vi "Fuel Injector Analysis Section.vi"(8 "error in (no error)":errorcluster, 11 "Node Ptr":T5 format="%.0x") -> (0 "error out":errorcluster)   [LabVIEW 2019, in "Fuel Injector Analysis Addon System Explorer.lvlib"]
uses:
  Fuel Injector Analysis Addon System Explorer.lvlib
  <vilib>/NI VeriStand/Custom Device API/Custom Device Item Ref.ctl
  Addon Shared/Types/Stage.PullIn.Types.ctl
  Addon Shared/Types/Stage.Transition.Types.ctl
  Types/Analysis.UI.Refs.ctl
  Addon Shared/Types/Analysis.Channels.Select.ctl
  <vilib>/NI VeriStand/Custom Device Tools/Custom Device Utility Library/Search Direction.ctl
  Addon Shared/SubVIs/Constants.vi
  <vilib>/NI VeriStand/Custom Device API/Set Item Property (U32).vi
  <vilib>/NI VeriStand/Custom Device API/Set Item Property (Variant).vi
  <vilib>/NI VeriStand/Custom Device API/Get Item Property (Variant).vi
  <vilib>/NI VeriStand/Custom Device API/Get Item Property (U32).vi
  <vilib>/NI VeriStand/Custom Device Tools/Custom Device Utility Library/NI VeriStand - Search for All Items by GUID.vi
  <vilib>/NI VeriStand/Custom Device Tools/Custom Device Utility Library/NI VeriStand - Search for Item by GUID.vi
  <vilib>/NI VeriStand/Custom Device API/Custom Device API.lvlib
  Addon Shared/Fuel Injector Analysis Addon Shared.lvlib
  <vilib>/NI VeriStand/Custom Device Tools/Custom Device Utility Library/Custom Device Utility Library.lvlib
panel:
  in  "Back":bool
  in  "Next":bool
  in  "Tab Control":T1(tab)
  in  "Path":path
  in  "Stages":string[](array[string])=["Boost", "Battery", "Off"]
  in  "Max Shots":T2(ring)=enum."1"
  out "Total Duration":dbl=1.0 caption="Total Event Duration" format="%#_p"
  in  "Pre-Trigger Samples":u8=1
  in  "Event Duration":dbl=1.0 format="%#_p"
  in  "Active Edge":bool=TRUE
  in  "Trigger Duration":dbl=1.0 caption="Trigger Duration (sec)" format="%#_p"
  in  "Initial Voltage Threshold":dbl=1.0 caption="Initial Voltage" format="%#_p"
  in  "Transitions":i32(listbox)
  in  "Pull In Type":T3
  in  "Stage Transition":T4
  in  "Level":dbl=1.0 format="%#_p"
  in  "Analysis":i32(listbox)=7
  in  "Stages List":i32(listbox)
  in  "Reset":bool
  in  "Apply":bool
  out "Injection":waveform(dbl)[](graph)
  out "Step":string
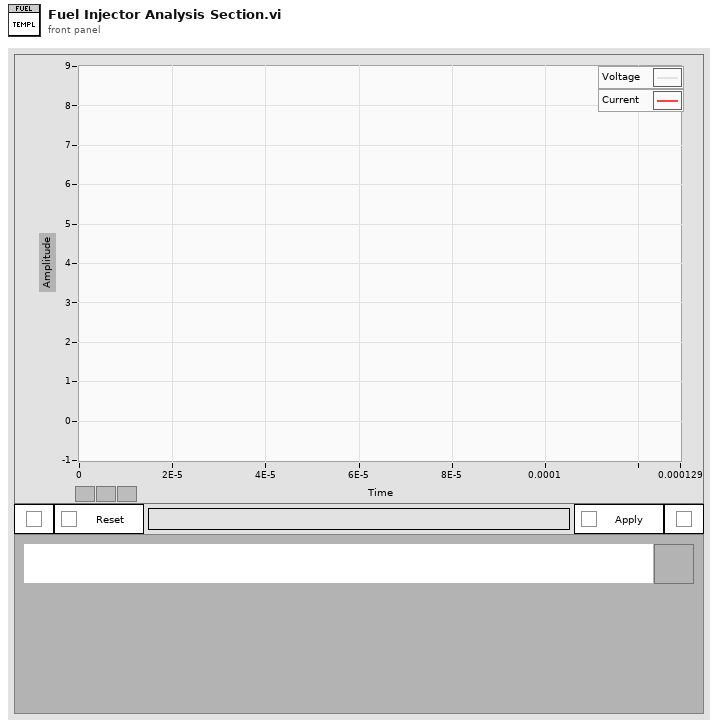
[diagram p1: front panel]
types:
  T1 = enum32{"Load Waveform", "Set Shots and Stages", "Set Event Duration", "Set Initial Voltage", "Set Stage Parsing Parameters", "Set Analysis Channels"}
  T2 = enum16{"0", "1", "2", "3", "4", "5", "6", "7", "8"}
  T3 = typedef "Fuel Injector Analysis Addon Shared.lvlib/Stage.PullIn.Types.ctl" = enum8{"Pull In Transition Pulses", "Pull In Transition Current Drop"}
  T4 = typedef "Fuel Injector Analysis Addon Shared.lvlib/Stage.Transition.Types.ctl" = enum8{"Stage Transition Inactive Time", "Stage Transition Voltage Increase", "Stage Transition Current Decrease", "Stage Transition Active Time"}
  T5 = typedef "Custom Device API.lvlib/Custom Device Item Ref.ctl" = u64
  T6 = typedef "Fuel Injector Analysis Addon System Explorer.lvlib/Analysis.UI.Refs.ctl" = cluster{"Path":refnum<vi>, "Pull In Transition":refnum<vi>, "Level":refnum<vi>, "Stage Transition":refnum<vi>, "Injection":refnum<vi>, "Tab":refnum<vi>, "Step":refnum<vi>, "Stages":refnum<vi>, "Transitions":refnum<vi>, "Initial Voltage":refnum<vi>, "Event Duration":refnum<vi>, "Max Shots":refnum<vi>, "Stages List":refnum<vi>, "Analysis":refnum<vi>, "Pre-Trigger Samples":refnum<vi>, "Trigger Duration":refnum<vi>, "dt":dbl, "Total Duration":refnum<vi>, "Next":refnum<vi>, "Back":refnum<vi>, "Active Edge":refnum<vi>}
  T7 = enum8{"Enabled", "Disabled", "Disabled and Grayed Out"}
  T8 = typedef "Fuel Injector Analysis Addon Shared.lvlib/Analysis.Channels.Select.ctl" = cluster{"Pull In Time":bool, "Pull In Max Current":bool, "Pull In Max Voltage":bool, "Pull In Min Voltage":bool, "Pull In Avg Voltage":bool, "Hold Time":bool, "Hold Max Current":bool, "Hold Min Current":bool, "Hold Avg Current":bool, "Hold Max Voltage":bool, "Hold Min Voltage":bool, "Hold Avg Max Voltage":bool, "Hold Avg Min Voltage":bool, "Off Time":bool, "Off Max Current":bool, "Off Min Current":bool, "Off Avg Current":bool, "Off Max Voltage":bool, "Off Min Voltage":bool, "Off Avg Voltage":bool, "Total Voltage Pulses":bool, "Total Stage Time":bool}
  T9 = typedef "Custom Device Utility Library.lvlib/Search Direction.ctl" = enum16{"Down", "Up"}
  T10 = typedef "Custom Device API.lvlib/Custom Device Commands.ctl" = enum16{"Default", "Item renamed", "Shutdown", "Dynamic button pressed"}
  T11 = typedef "LVPoint32TypeDef.ctl" = cluster{"Horizontal":i32, "Vertical":i32}
  T12 = typedef "LVCursorListTypeDef.ctl" = cluster{"Name":string, "Color":u32, "Style":u8, "Point Style":u8, "Name Visible":bool, "Allow Drag":bool, "Cursor Mode":u32, "Plot":i32, "Index":i32, "Position":cluster{"X":dbl, "Y":dbl}, "X Scale":u32, "Y Scale":u32, "Watch Plots":i32[], "Watch All Plots":bool, "Plot Area":i32, "Label Offset":cluster{"X":dbl, "Y":dbl}}[]
  T13 = cluster{"Name":string, "Color":u32, "Style":u8, "Point Style":u8, "Name Visible":bool, "Allow Drag":bool, "Cursor Mode":u32, "Plot":i32, "Index":i32, "Position":cluster{"X":dbl, "Y":dbl}, "X Scale":u32, "Y Scale":u32, "Watch Plots":i32[], "Watch All Plots":bool, "Plot Area":i32, "Label Offset":cluster{"X":dbl, "Y":dbl}}
  T14 = typedef "Custom Device API.lvlib/Custom Device Channel.ctl" = cluster{"Type":T15, "Units":string, "Default Value":dbl, "Faultable":bool, "Scalable":bool}
  T15 = typedef "Custom Device API.lvlib/Custom Device Channel Type.ctl" = enum16{"Input", "Output"}
  T16 = typedef "Custom Device API.lvlib/Custom Device Item Info.ctl" = cluster{"Name":string, "Is Channel":bool, "GUID":string, "Is Waveform":bool}
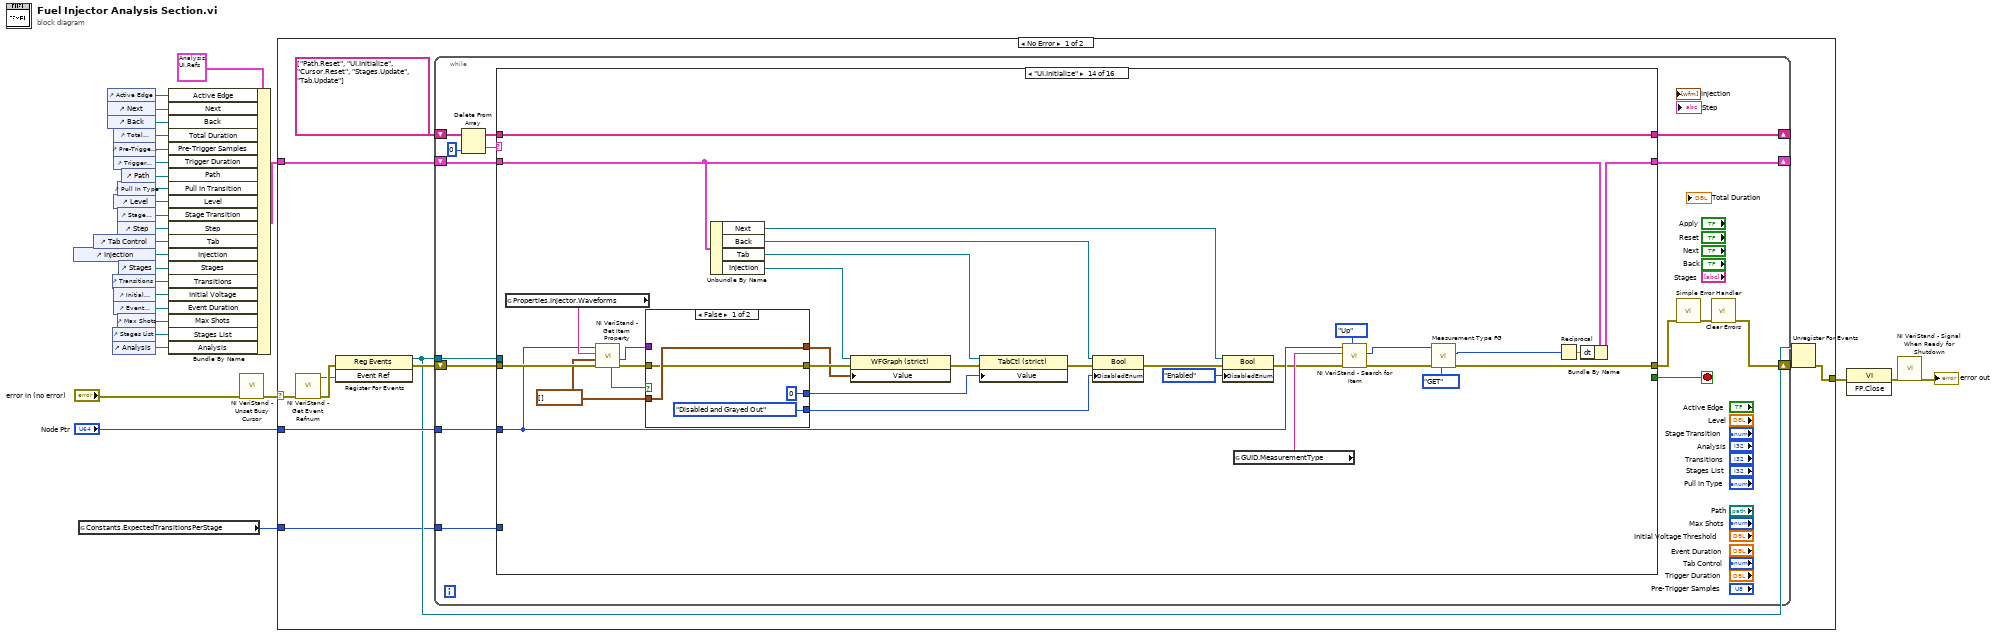
[diagram p0: block diagram]
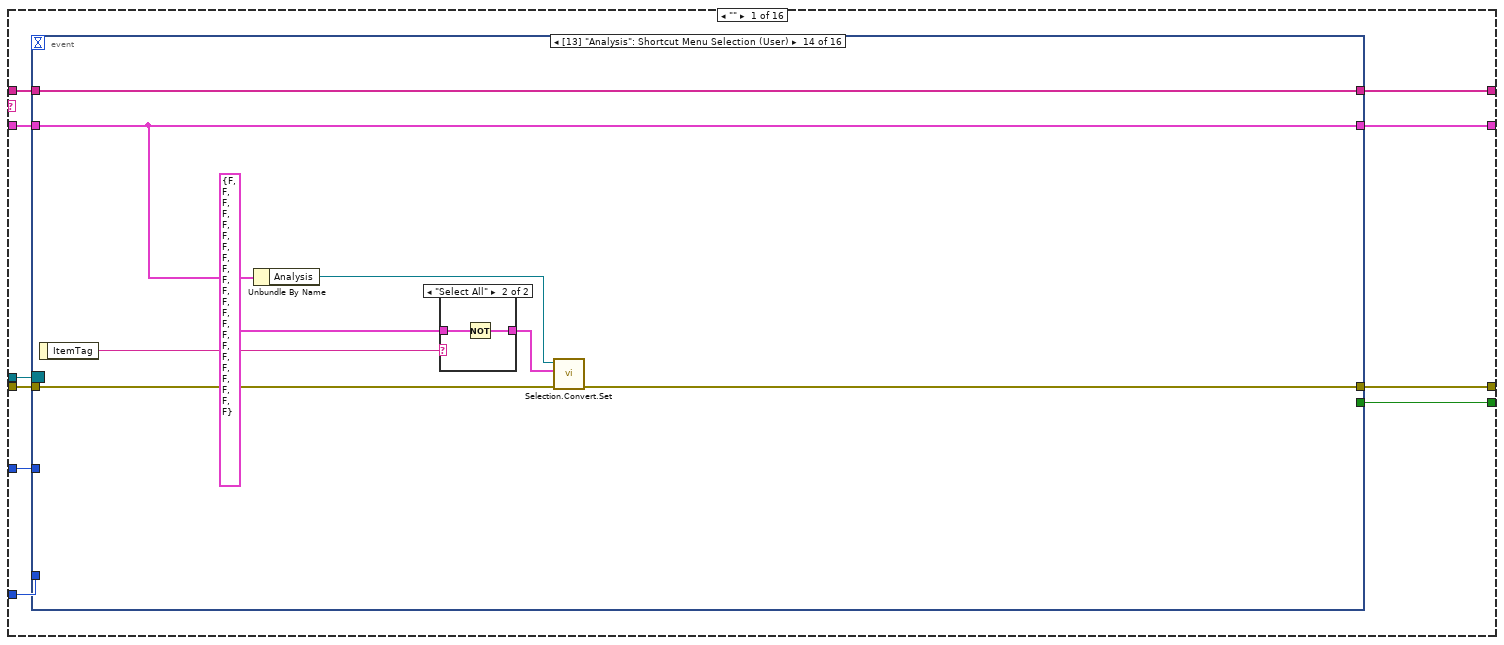
[diagram p2: hidden frame]
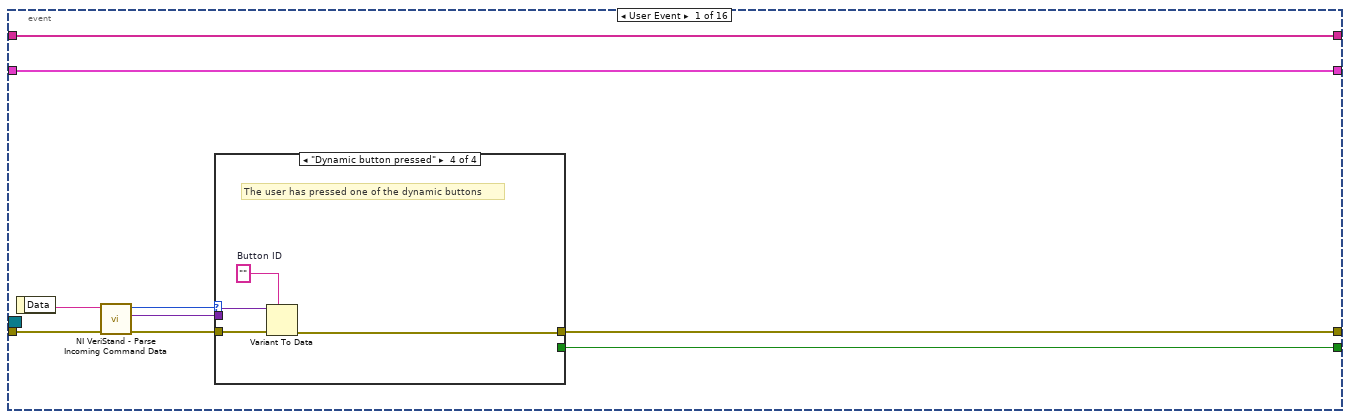
[diagram p3: hidden frame]
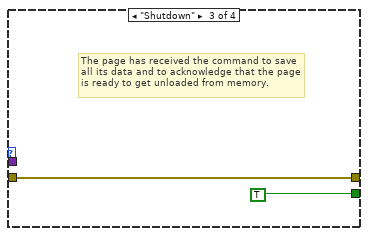
[diagram p6: hidden frame]
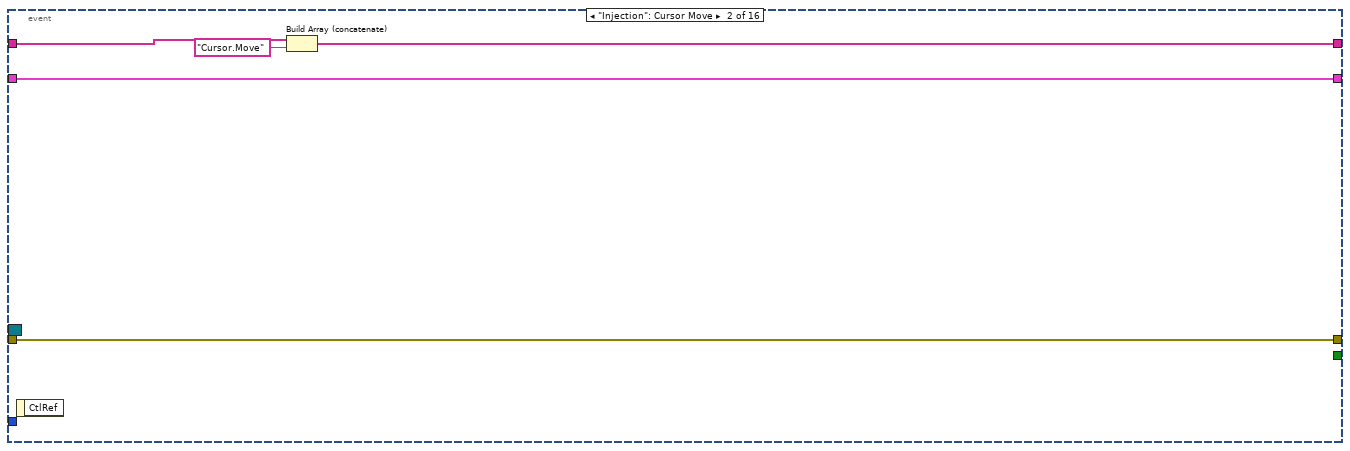
[diagram p7: hidden frame]
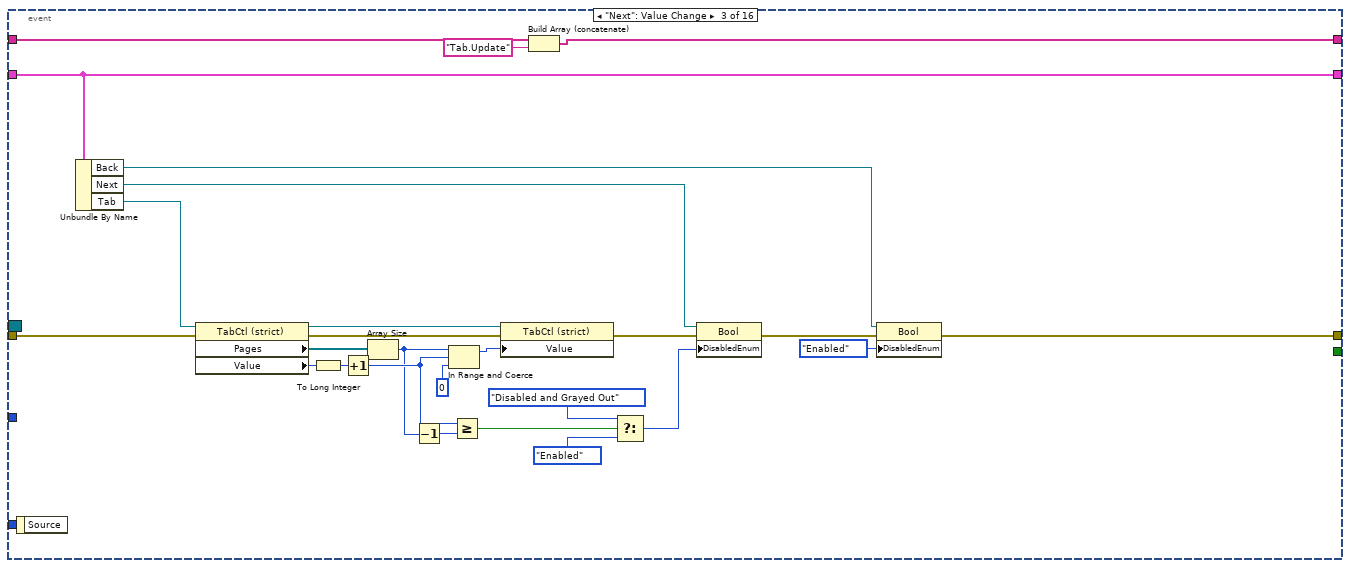
[diagram p8: hidden frame]
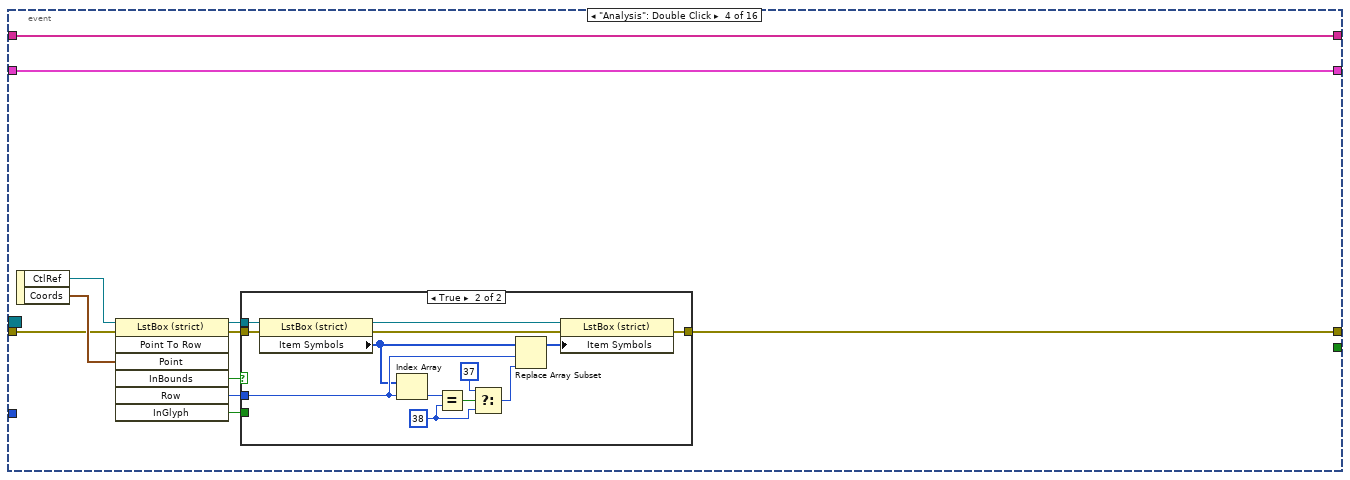
[diagram p9: hidden frame]
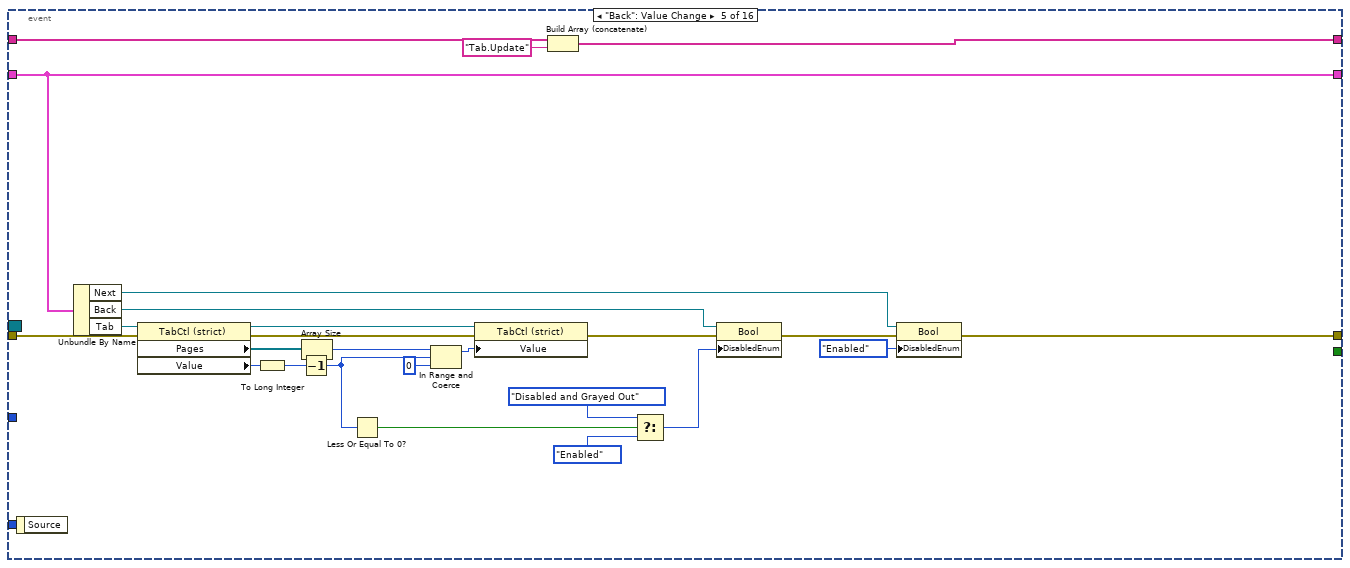
[diagram p11: hidden frame]
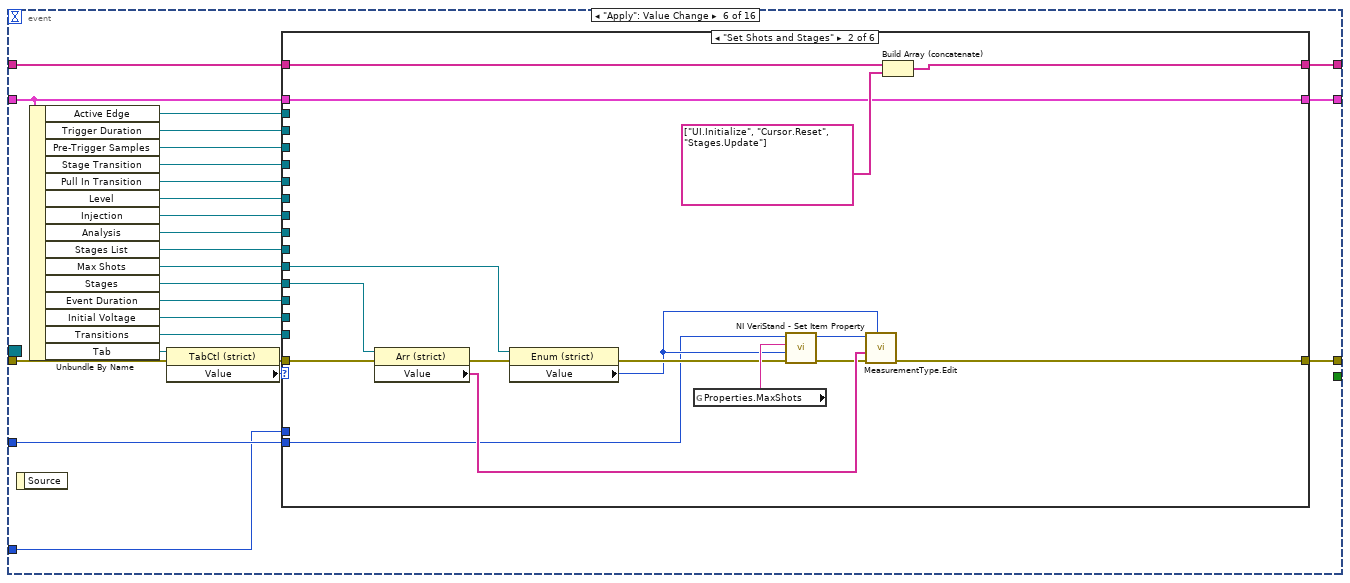
[diagram p12: hidden frame]
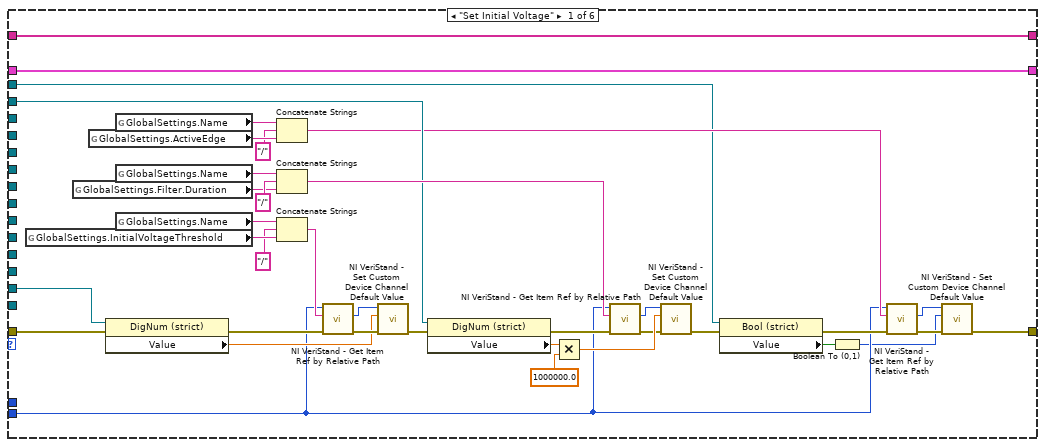
[diagram p13: hidden frame]
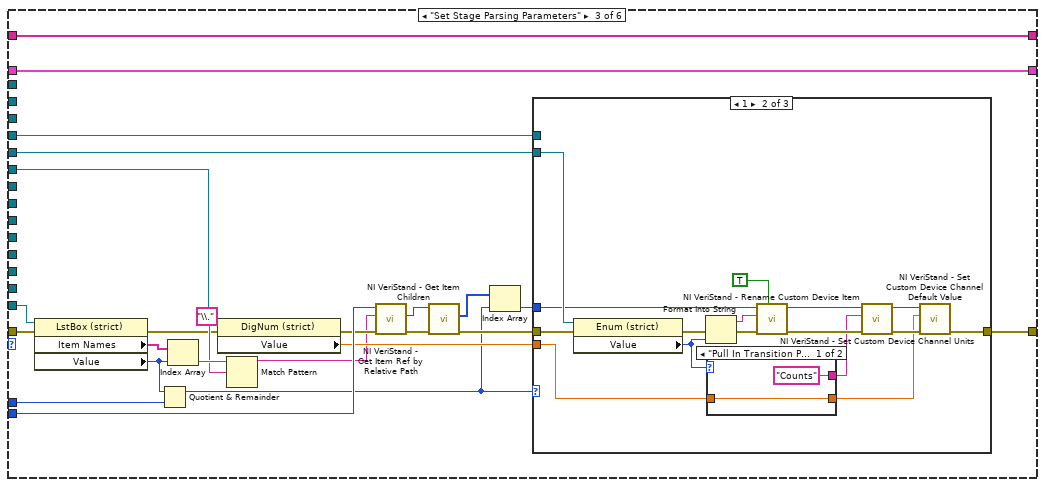
[diagram p14: hidden frame]
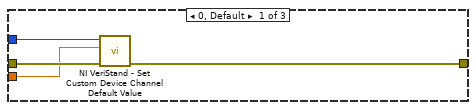
[diagram p15: hidden frame]
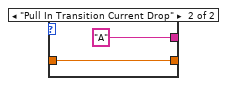
[diagram p16: hidden frame]
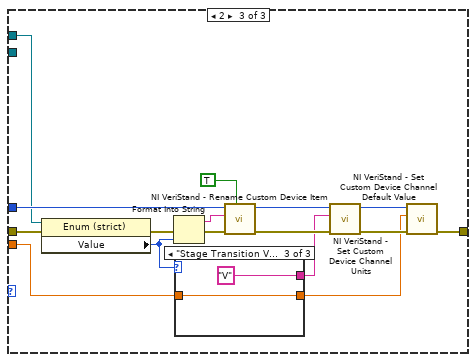
[diagram p17: hidden frame]
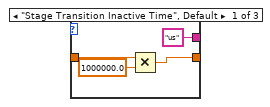
[diagram p18: hidden frame]
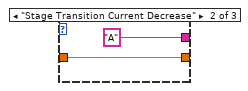
[diagram p19: hidden frame]
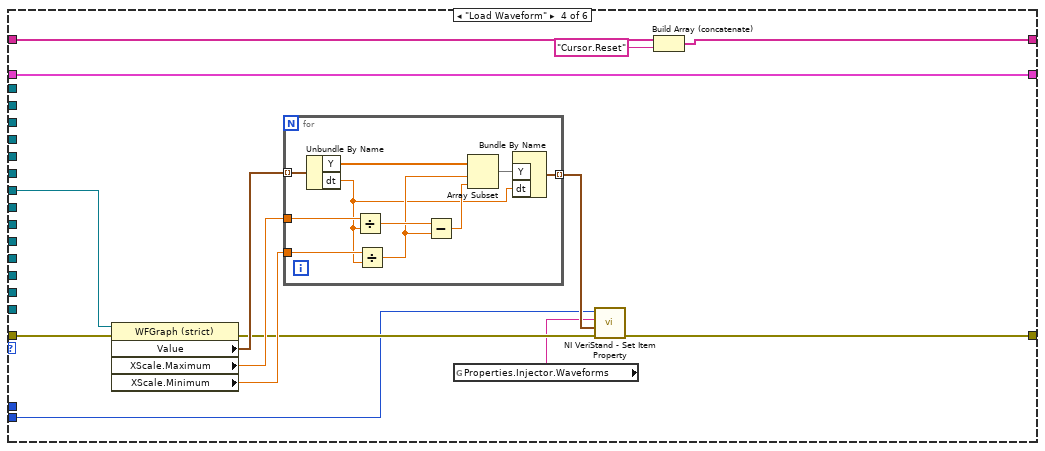
[diagram p20: hidden frame]
diagram:
  n1 = control-ref of="Injection"() -> (w21:refnum<vi>)
  n2 = global read "Constants.vi" "Constants.ExpectedTransitionsPerStage"() -> (w7:u32)
  n3 = control-ref of="Tab Control"() -> (w10:refnum<vi>)
  n4 = control-ref of="Active Edge"() -> (w1:refnum<vi>)
  n5 = control-ref of="Next"() -> (w3:refnum<vi>)
  n6 = control-ref of="Back"() -> (w2:refnum<vi>)
  n7 = control-ref of="Transitions"() -> (w16:refnum<vi>)
  n8 = control-ref of="Stages List"() -> (w12:refnum<vi>)
  n9 = control-ref of="Analysis"() -> (w11:refnum<vi>)
  n10 = control-ref of="Total Duration"() -> (w4:refnum<vi>)
  n11 = control-ref of="Pre-Trigger Samples"() -> (w5:refnum<vi>)
  n12 = control-ref of="Trigger Duration"() -> (w6:refnum<vi>)
  n13 = control-ref of="Level"() -> (w20:refnum<vi>)
  n14 = control-ref of="Initial Voltage Threshold"() -> (w15:refnum<vi>)
  n15 = control-ref of="Event Duration"() -> (w14:refnum<vi>)
  n16 = control-ref of="Pull In Type"() -> (w9:refnum<vi>)
  n17 = control-ref of="Stage Transition"() -> (w8:refnum<vi>)
  n18 = control-ref of="Step"() -> (w18:refnum<vi>)
  n19 = control-ref of="Max Shots"() -> (w13:refnum<vi>)
  n20 = control-ref of="Stages"() -> (w17:refnum<vi>)
  n21 = control-ref of="Path"() -> (w19:refnum<vi>)
  n22 = Bundle By Name(cluster=T6 {"Path"=refnum, "Pull In Transition"=refnum, "Level"=refnum, "Stage Transition"=refnum, "Injection"=refnum, "Tab"=refnum, "Step"=refnum, "Stages"=refnum, "Transitions"=refnum, "Initial Voltage"=refnum, "Event Duration"=refnum, "Max Shots"=refnum, "Stages List"=refnum, "Analysis"=refnum, "Pre-Trigger Samples"=refnum, "Trigger Duration"=refnum, "dt"=0.0, "Total Duration"=refnum, "Next"=refnum, "Back"=refnum, "Active Edge"=refnum}, "Active Edge"=w1, "Next"=w3, "Back"=w2, "Total Duration"=w4, "Pre-Trigger Samples"=w5, "Trigger Duration"=w6, "Path"=w19, "Pull In Transition"=w9, "Level"=w20, "Stage Transition"=w8, "Step"=w18, "Tab"=w10, "Injection"=w21, "Stages"=w17, "Transitions"=w16, "Initial Voltage"=w15, "Event Duration"=w14, "Max Shots"=w13, "Stages List"=w12, "Analysis"=w11) -> (w23:T6)
  n23 = call <vilib>:"NI VeriStand - Unset Busy Cursor.vi"("error in (no error)"="error in (no error)") -> ("error out"=w25:errorcluster)  [unwired: 10 out]
  n24 = case shown="No Error" w25 {
    selector: w25 -> [w34 w1059]
    tunnel: [w38 w1057] -> w29
    tunnel: "Node Ptr" -> [w35 _]
    tunnel: w23 -> [w33 _]
    tunnel: w7 -> [w30 _]
    frame No Error {
      n25 = call <vilib>:"NI VeriStand - Get Event Refnum.vi"("error in (no error)"=w34) -> ("error out"=w40:errorcluster, "Event Ref"=w37:refnum<user-event>)  [unwired: 9 out]
      n26 = register-events(error in=w40, w37) -> (reference out=w31:refnum<event-registration>, error out=w36:errorcluster)  [unwired: 1 in]
      n27 = while {
        tunnel: w35 -> [w53]
        shift-right: [w50] -> w39
        shift-left: w36 -> [w55]
        shift-right: [w43] -> _
        shift-left: string[] ["Path.Reset", "UI.Initialize", "Cursor.Reset", "Stages.Update", "Tab.Update"] -> [w48]
        tunnel: w31 -> [w44]
        tunnel: w30 -> [w42]
        shift-right: [w41] -> _
        shift-left: w33 -> [w49]
        stop <- w54 stop-if-true
        n28 = Delete From Array(array=w48, index=0) -> (deleted portion=w46:string, array with subset deleted=w45:string[])  [unwired: 1 in]
        n29 = case shown="\"UI.Initialize\"" w46 {
          tunnel: w55 -> [w65 w470 w505 w632 w645 w659 w676 w716 w760 w776 w811 w855 w878 w1029 w1050 w1056]
          tunnel: w44 -> [w64 _ _ _ _ _ _ _ _ _ _ _ _ _ _ _]
          tunnel: [w63 _ _ _ _ _ _ _ _ _ _ _ _ _ _ _] -> w54
          tunnel: w53 -> [w62 w469 w498 _ _ _ w677 w693 w744 w774 _ _ w877 w1022 _ _]
          tunnel: [w61 w471 w503 w633 w644 w658 w673 w696 w734 w770 w819 w854 w876 w1018 w1050 w1053] -> w52
          tunnel: w49 -> [w60 w472 w504 w640 w647 w661 w684 w715 w759 w791 w805 w866 w868 w1015 w1048 w1054]
          tunnel: w45 -> [w59 w481 w495 w634 w653 w667 w672 w707 w767 w787 w817 w867 w874 w1027 w1049 w1055]
          tunnel: [w58 w481 w494 w634 w653 w667 w672 w706 w754 w787 w818 w867 w873 w1027 w1049 w1055] -> w43
          tunnel: w42 -> [w57 _ w497 _ _ _ _ _ _ _ _ _ w871 _ _ _]
          tunnel: [w56 w472 w504 w640 w647 w661 w684 w715 w759 w791 w806 w866 w869 w1014 w1048 w1054] -> w41
          frame "" {
            n30 = event shown="[13] \"Analysis\": Shortcut Menu Selection (User)" {
              selector: w64 -> [_ _ _ _ _ _ _ _ _ _ _ _ _ _ _ _]
              dyn-events: _ -> [_ _ _ _ _ _ _ _ _ _ _ _ _ _ _ _]
              timeout: _ -> [_ _ _ _ _ _ _ _ _ _ _ _ _ _ _ _]
              tunnel: w65 -> [w74 w84 w113 w116 w163 w188 w380 w387 w390 w395 w404 w417 w440 w453 w460 w465]
              tunnel: [w70 _ _ _ _ _ _ _ _ _ _ _ _ _ _ _] -> w63
              tunnel: [w69 w84 w98 w115 w145 w182 w380 w387 w390 w395 w402 w413 w439 w450 w460 w465] -> w61
              tunnel: w62 -> [_ _ _ _ _ w183 _ _ _ _ _ _ _ _ _ _]
              tunnel: w60 -> [w66 w83 w108 w114 w158 w165 w379 w384 w389 w394 w405 w418 w431 w452 w461 w466]
              tunnel: w59 -> [w67 w87 w105 w124 w156 w177 w383 w388 w393 w398 w400 w415 w435 w454 w462 w467]
              tunnel: [w67 w86 w104 w124 w155 w176 w382 w386 w392 w397 w399 w414 w434 w454 w459 w464] -> w58
              tunnel: w57 -> [_ _ _ _ _ w169 _ _ _ _ _ _ _ _ _ _]
              tunnel: [w66 w83 w108 w114 w158 w166 w379 w384 w389 w394 w405 w418 w431 w452 w461 w466] -> w56
              event User Event {
                n31 = event-data() -> ("Data"=w73:string)  [unwired: 1 out]
                n32 = call <vilib>:"NI VeriStand - Parse Incoming Command Data.vi"("error in (no error)"=w74, "Incoming data"=w73) -> ("error out"=w72:errorcluster, "Outgoing data"=w68:variant, "Action"=w71:T10)  [unwired: 7 out]
                n33 = case shown="\"Dynamic button pressed\"" w71 {
                  tunnel: w72 -> [w75 w76 w77 w82]
                  tunnel: [_ _ TRUE _] -> w70
                  tunnel: [w75 w76 w77 w79] -> w69
                  tunnel: w68 -> [_ _ _ w81]
                  frame "Default", Default {
                  }
                  frame "Item renamed" {
                  }
                  frame "Shutdown" {
                    # "The page has received the command to save all its data and to acknowledge that the page is ready to get unloaded from memory."
                  }
                  frame "Dynamic button pressed" {
                    w80 = ""  # Button ID
                    # "The user has pressed one of the dynamic buttons"
                    n34 = Variant To Data(error in=w82, type=w80, Variant=w81) -> (error out=w79:errorcluster)  [unwired: 1 out]
                  }
                }
              }
              event "Injection": Cursor Move {
                n35 = event-data() -> ()  [unwired: 2 out]
                n36 = Build Array (concatenate)(w87, "Cursor.Move") -> (w86:string[])
              }
              event "Next": Value Change {
                n37 = event-data() -> ()  [unwired: 2 out]
                n38 = Unbundle By Name(w108) -> ("Back"=w96:refnum<vi>, "Next"=w97:refnum<vi>, "Tab"=w107:refnum<vi>)
                n39 = property class="TabCtl (strict)"(reference=w107, error in=w113) -> (reference out=w110:refnum<vi>, error out=w103:errorcluster, "Pages"=w112:refnum<vi>[], "Value"=w111:T1)
                n40 = To Long Integer(number=w111) -> (32bit integer=w102:i32)
                n41 = Increment(x=w102) -> (x+1=w90:i32)
                n42 = Array Size(array=w112) -> (size(s)=w89:i32)
                n43 = Decrement(x=w89) -> (x-1=w88:i32)
                n44 = In Range and Coerce(upper limit=w89, x=w90, lower limit=0) -> (coerced(x)=w109:i32)  [unwired: 1 out]
                n45 = Greater Or Equal?(x=w90, y=w88) -> (x >= y?=w94:bool)
                n46 = property class="TabCtl (strict)"(reference=w110, error in=w103, "Value"=w109) -> (error out=w99:errorcluster)  [unwired: 1 out]
                n47 = Build Array (concatenate)(w105, "Tab.Update") -> (w104:string[])
                n48 = Select(t=T7."Disabled and Grayed Out" ("Disabled"), s=w94, f=T7."Enabled" ("Disabled")) -> (s? t:f=w91:T7)
                n49 = property class="Bool"(reference=w97, error in=w99, "DisabledEnum"=w91) -> (error out=w100:errorcluster)  [unwired: 1 out]
                n50 = property class="Bool"(reference=w96, error in=w100, "DisabledEnum"=T7."Enabled" ("Disabled")) -> (error out=w98:errorcluster)  [unwired: 1 out]
              }
              event "Analysis": Double Click {
                n51 = event-data() -> ("CtlRef"=w118:refnum<vi>, "Coords"=w117:T11)  [unwired: 1 out]
                n52 = invoke class="LstBox (strict)" method="Point To Row"(reference=w118, error in=w116, "Point"=w117) -> (reference out=w122:refnum<vi>, error out=w121:errorcluster, "InBounds"=w119:bool, "Row"=w120:i32, "InGlyph"=w123:bool)  [unwired: 4 in, 2 out]
                n53 = case shown="True" w119 {
                  tunnel: w123 -> [_ _]
                  tunnel: w122 -> [_ w138]
                  tunnel: w121 -> [w125 w137]
                  tunnel: w120 -> [_ w136]
                  tunnel: [w125 w126] -> w115
                  frame False {
                  }
                  frame True {
                    w133 = 38
                    n54 = property class="LstBox (strict)"(reference=w138, error in=w137) -> (reference out=w129:refnum<vi>, error out=w128:errorcluster, "Item Symbols"=w131:i32[])
                    n55 = Index Array(array=w131, index=w136) -> (element=w135:i32)
                    n56 = Equal?(x=w135, y=w133) -> (x = y?=w134:bool)
                    n57 = Select(t=37, s=w134, f=w133) -> (s? t:f=w130:i32)
                    n58 = Replace Array Subset(array=w131, new element=w130, index=w136) -> (w127:i32[])
                    n59 = property class="LstBox (strict)"(reference=w129, error in=w128, "Item Symbols"=w127) -> (error out=w126:errorcluster)  [unwired: 1 out]
                  }
                }
              }
              event "Back": Value Change {
                n60 = event-data() -> ()  [unwired: 2 out]
                n61 = Unbundle By Name(w158) -> ("Next"=w143:refnum<vi>, "Back"=w144:refnum<vi>, "Tab"=w157:refnum<vi>)
                n62 = property class="TabCtl (strict)"(reference=w157, error in=w163) -> (reference out=w160:refnum<vi>, error out=w153:errorcluster, "Pages"=w162:refnum<vi>[], "Value"=w161:T1)
                n63 = To Long Integer(number=w161) -> (32bit integer=w152:i32)
                n64 = Decrement(x=w152) -> (x-1=w140:i32)
                n65 = Array Size(array=w162) -> (size(s)=w141:i32)
                n66 = Less Or Equal To 0?(x=w140) -> (x <= 0?=w139:bool)
                n67 = In Range and Coerce(upper limit=w141, x=w140, lower limit=0) -> (coerced(x)=w159:i32)  [unwired: 1 out]
                n68 = property class="TabCtl (strict)"(reference=w160, error in=w153, "Value"=w159) -> (error out=w146:errorcluster)  [unwired: 1 out]
                n69 = Build Array (concatenate)(w156, "Tab.Update") -> (w155:string[])
                n70 = Select(t=T7."Disabled and Grayed Out" ("Disabled"), s=w139, f=T7."Enabled" ("Disabled")) -> (s? t:f=w147:T7)
                n71 = property class="Bool"(reference=w144, error in=w146, "DisabledEnum"=w147) -> (error out=w151:errorcluster)  [unwired: 1 out]
                n72 = property class="Bool"(reference=w143, error in=w151, "DisabledEnum"=T7."Enabled" ("Disabled")) -> (error out=w145:errorcluster)  [unwired: 1 out]
              }
              event "Apply": Value Change {
                n73 = event-data() -> ()  [unwired: 2 out]
                n74 = Unbundle By Name(w165) -> ("Active Edge"=w164:refnum<vi>, "Trigger Duration"=w167:refnum<vi>, "Pre-Trigger Samples"=w168:refnum<vi>, "Stage Transition"=w172:refnum<vi>, "Pull In Transition"=w173:refnum<vi>, "Level"=w174:refnum<vi>, "Injection"=w175:refnum<vi>, "Analysis"=w178:refnum<vi>, "Stages List"=w179:refnum<vi>, "Max Shots"=w180:refnum<vi>, "Stages"=w181:refnum<vi>, "Event Duration"=w184:refnum<vi>, "Initial Voltage"=w185:refnum<vi>, "Transitions"=w170:refnum<vi>, "Tab"=w187:refnum<vi>)
                n75 = property class="TabCtl (strict)"(reference=w187, error in=w188) -> (error out=w186:errorcluster, "Value"=w171:T1)  [unwired: 1 out]
                n76 = case shown="\"Set Shots and Stages\"" w171 {
                  tunnel: w186 -> [w222 w241 w264 w327 w352 w354]
                  tunnel: w185 -> [w221 _ _ _ _ _]
                  tunnel: [w193 w231 w256 w320 w341 w355] -> w182
                  tunnel: w184 -> [_ _ _ _ _ w375]
                  tunnel: w183 -> [w191 w230 w260 w318 w348 w360]
                  tunnel: w181 -> [_ w238 _ _ _ _]
                  tunnel: w180 -> [_ w237 _ _ _ _]
                  tunnel: w179 -> [_ _ _ _ w351 _]
                  tunnel: w178 -> [_ _ _ _ w343 _]
                  tunnel: w177 -> [w215 w236 w265 w326 w340 w369]
                  tunnel: [w215 w235 w265 w316 w340 w369] -> w176
                  tunnel: w175 -> [_ _ _ w325 _ _]
                  tunnel: w174 -> [_ _ w253 _ _ _]
                  tunnel: w173 -> [_ _ w251 _ _ _]
                  tunnel: w172 -> [_ _ w250 _ _ _]
                  tunnel: w170 -> [_ _ w244 _ _ _]
                  tunnel: w169 -> [_ _ w243 _ _ _]
                  tunnel: w168 -> [_ _ _ _ _ w358]
                  tunnel: w167 -> [w207 _ _ _ _ _]
                  tunnel: [w203 w228 w242 w314 w338 w356] -> w166
                  tunnel: w165 -> [w203 w228 w242 w314 w338 w356]
                  tunnel: w164 -> [w190 _ _ _ _ _]
                  frame "Set Initial Voltage" {
                    n77 = global read "Constants.vi" "GlobalSettings.InitialVoltageThreshold"() -> (w224:string)
                    n78 = global read "Constants.vi" "GlobalSettings.Filter.Duration"() -> (w210:string)
                    n79 = global read "Constants.vi" "GlobalSettings.ActiveEdge"() -> (w201:string)
                    n80 = property class="DigNum (strict)"(reference=w221, error in=w222) -> (error out=w218:errorcluster, "Value"=w217:dbl)  [unwired: 1 out]
                    n81 = global read "Constants.vi" "GlobalSettings.Name"() -> (w202:string)
                    n82 = global read "Constants.vi" "GlobalSettings.Name"() -> (w209:string)
                    n83 = global read "Constants.vi" "GlobalSettings.Name"() -> (w225:string)
                    n84 = Concatenate Strings(w202, "/" ("string"), w201) -> (w192:string)
                    n85 = Concatenate Strings(w209, "/" ("string"), w210) -> (w214:string)
                    n86 = Concatenate Strings(w225, "/" ("string"), w224) -> (w216:string)
                    n87 = call <vilib>:"NI VeriStand - Get Item Ref by Relative Path.vi"("error in"=w218, "Relative Item Path"=w216, "Section Ref in"=w191) -> ("error out"=w220:errorcluster, "Item Ref"=w219:T5)  [unwired: 5 in, 2 out]
                    n88 = call <vilib>:"NI VeriStand - Set Custom Device Channel Default Value.vi"("error in (no error)"=w220, "Default Value"=w217, "Channel Ref in"=w219) -> ("error out"=w208:errorcluster)  [unwired: 7 in, 1 out]
                    n89 = property class="DigNum (strict)"(reference=w207, error in=w208) -> (error out=w213:errorcluster, "Value"=w205:dbl)  [unwired: 1 out]
                    n90 = Multiply(x=w205, y=1000000.0) -> (x*y=w204:dbl)
                    n91 = call <vilib>:"NI VeriStand - Get Item Ref by Relative Path.vi"("error in"=w213, "Relative Item Path"=w214, "Section Ref in"=w191) -> ("error out"=w196:errorcluster, "Item Ref"=w212:T5)  [unwired: 5 in, 2 out]
                    n92 = call <vilib>:"NI VeriStand - Set Custom Device Channel Default Value.vi"("error in (no error)"=w196, "Default Value"=w204, "Channel Ref in"=w212) -> ("error out"=w195:errorcluster)  [unwired: 7 in, 1 out]
                    n93 = property class="Bool (strict)"(reference=w190, error in=w195) -> (error out=w194:errorcluster, "Value"=w199:bool)  [unwired: 1 out]
                    n94 = Boolean To (0,1)(Boolean=w199) -> (0, 1=w189:i16)
                    n95 = call <vilib>:"NI VeriStand - Get Item Ref by Relative Path.vi"("error in"=w194, "Relative Item Path"=w192, "Section Ref in"=w191) -> ("error out"=w197:errorcluster, "Item Ref"=w198:T5)  [unwired: 5 in, 2 out]
                    n96 = call <vilib>:"NI VeriStand - Set Custom Device Channel Default Value.vi"("error in (no error)"=w197, "Default Value"=w189, "Channel Ref in"=w198) -> ("error out"=w193:errorcluster)  [unwired: 7 in, 1 out]
                  }
                  frame "Set Shots and Stages" {
                    n97 = property class="Arr (strict)"(reference=w238, error in=w241) -> (error out=w240:errorcluster, "Value"=w239:string[])  [unwired: 1 out]
                    n98 = property class="Enum (strict)"(reference=w237, error in=w240) -> (error out=w233:errorcluster, "Value"=w232:T2)  [unwired: 1 out]
                    n99 = global read "Constants.vi" "Properties.MaxShots"() -> (w234:string)
                    n100 = call-poly <vilib>:"NI VeriStand - Set Item Property.vi"("error in (no error)"=w233, "Value"=w232, "Property Name"=w234, "Item Ref in"=w230) -> ("error out"=w227:errorcluster, "Item Ref out"=w226:T5)  [unwired: 5 in, 1 out]
                    n101 = call "MeasurementType.Edit.vi"("Max Shots"=w232, "error in (no error)"=w227, "Stages"=w239, "Item Ref in"=w226) -> ("error out"=w231:errorcluster)  [unwired: 7 in]
                    n102 = Build Array (concatenate)(w236, string[] ["UI.Initialize", "Cursor.Reset", "Stages.Update"]) -> (w235:string[])
                  }
                  frame "Set Stage Parsing Parameters" {
                    n103 = property class="LstBox (strict)"(reference=w244, error in=w264) -> (error out=w255:errorcluster, "Item Names"=w263:string[], "Value"=w252:i32)  [unwired: 1 out]
                    n104 = Quotient & Remainder(x=w252, y=w243) -> (x-y*floor(x/y)=w246:u32)  [unwired: 1 out]
                    n105 = Index Array(array=w263, index=w252) -> (element=w262:string)
                    n106 = property class="DigNum (strict)"(reference=w253, error in=w255) -> (error out=w254:errorcluster, "Value"=w247:dbl)  [unwired: 1 out]
                    n107 = Match Pattern(string=w262, regular expression="\\.") -> (before substring=w245:string)  [unwired: 1 in, 3 out]
                    n108 = call <vilib>:"NI VeriStand - Get Item Ref by Relative Path.vi"("error in"=w254, "Relative Item Path"=w245, "Section Ref in"=w260) -> ("error out"=w259:errorcluster, "Item Ref"=w258:T5)  [unwired: 5 in, 2 out]
                    n109 = call <vilib>:"NI VeriStand - Get Item Children.vi"("error in (no error)"=w259, "Item Ref in"=w258) -> ("error out"=w249:errorcluster, "Child Refs"=w257:T5[])  [unwired: 6 in, 2 out]
                    n110 = Index Array(array=w257, index=w246) -> (element=w248:T5)
                    n111 = case shown="1" w246 {
                      tunnel: w249 -> [w269 w278 w305]
                      tunnel: [w267 w276 w294] -> w256
                      tunnel: w248 -> [w268 w271 w301]
                      tunnel: w251 -> [_ w285 _]
                      tunnel: w250 -> [_ _ w296]
                      tunnel: w247 -> [w266 w273 w291]
                      frame 0, Default {
                        n112 = call <vilib>:"NI VeriStand - Set Custom Device Channel Default Value.vi"("error in (no error)"=w269, "Default Value"=w266, "Channel Ref in"=w268) -> ("error out"=w267:errorcluster)  [unwired: 7 in, 1 out]
                      }
                      frame 1 {
                        n113 = property class="Enum (strict)"(reference=w285, error in=w278) -> (error out=w284:errorcluster, "Value"=w280:T3)  [unwired: 1 out]
                        n114 = Format Into String(error in=w284, w280) -> (resulting string=w270:string, error out=w283:errorcluster)  [unwired: 2 in]
                        n115 = case shown="\"Pull In Transition Pulses\", Default" w280 {
                          tunnel: ["Counts" "A"] -> w279
                          tunnel: [w286 w288] -> w274
                          tunnel: w273 -> [w286 w288]
                          frame "Pull In Transition Pulses", Default {
                          }
                          frame "Pull In Transition Current Drop" {
                          }
                        }
                        n116 = call <vilib>:"NI VeriStand - Rename Custom Device Item.vi"("Force Rename (F)"=TRUE, "error in (no error)"=w283, "New Name"=w270, "Item Ref in"=w271) -> ("error out"=w282:errorcluster, "Item Ref out"=w281:T5)  [unwired: 5 in, 1 out]
                        n117 = call <vilib>:"NI VeriStand - Set Custom Device Channel Units.vi"("error in (no error)"=w282, "Units"=w279, "Channel Ref in"=w281) -> ("error out"=w277:errorcluster, "Channel Ref out"=w275:T5)  [unwired: 7 in]
                        n118 = call <vilib>:"NI VeriStand - Set Custom Device Channel Default Value.vi"("error in (no error)"=w277, "Default Value"=w274, "Channel Ref in"=w275) -> ("error out"=w276:errorcluster)  [unwired: 7 in, 1 out]
                      }
                      frame 2 {
                        n119 = property class="Enum (strict)"(reference=w296, error in=w305) -> (error out=w304:errorcluster, "Value"=w298:T4)  [unwired: 1 out]
                        n120 = Format Into String(error in=w304, w298) -> (resulting string=w303:string, error out=w302:errorcluster)  [unwired: 2 in]
                        n121 = case shown="\"Stage Transition Voltage Increase\"" w298 {
                          tunnel: ["us" "A" "V"] -> w297
                          tunnel: [w307 w310 w312] -> w292
                          tunnel: w291 -> [w308 w310 w312]
                          frame "Stage Transition Inactive Time", Default {
                            n122 = Multiply(x=w308, y=1000000.0) -> (x*y=w307:dbl)
                          }
                          frame "Stage Transition Current Decrease" {
                          }
                          frame "Stage Transition Voltage Increase" {
                          }
                        }
                        n123 = call <vilib>:"NI VeriStand - Rename Custom Device Item.vi"("Force Rename (F)"=TRUE, "error in (no error)"=w302, "New Name"=w303, "Item Ref in"=w301) -> ("error out"=w300:errorcluster, "Item Ref out"=w299:T5)  [unwired: 5 in, 1 out]
                        n124 = call <vilib>:"NI VeriStand - Set Custom Device Channel Units.vi"("error in (no error)"=w300, "Units"=w297, "Channel Ref in"=w299) -> ("error out"=w295:errorcluster, "Channel Ref out"=w293:T5)  [unwired: 7 in]
                        n125 = call <vilib>:"NI VeriStand - Set Custom Device Channel Default Value.vi"("error in (no error)"=w295, "Default Value"=w292, "Channel Ref in"=w293) -> ("error out"=w294:errorcluster)  [unwired: 7 in, 1 out]
                      }
                    }
                  }
                  frame "Load Waveform" {
                    n126 = property class="WFGraph (strict)"(reference=w325, error in=w327) -> (error out=w321:errorcluster, "Value"=w324:waveform(dbl)[], "XScale.Maximum"=w323:dbl, "XScale.Minimum"=w322:dbl)  [unwired: 1 out]
                    n127 = for {
                      tunnel: w324 -> [w337] mode=indexing
                      tunnel: w323 -> [w336]
                      tunnel: w322 -> [w335]
                      tunnel: [w328] -> w319 mode=indexing
                      n128 = Unbundle By Name(w337) -> ("Y"=w333:dbl[], "dt"=w329:dbl)
                      n129 = Divide(x=w336, y=w329) -> (x/y=w334:dbl)
                      n130 = Divide(x=w335, y=w329) -> (x/y=w332:dbl)
                      n131 = Subtract(x=w334, y=w332) -> (x-y=w331:dbl)
                      n132 = Array Subset(array=w333, index=w332, length=w331) -> (w330:dbl[])
                      n133 = Bundle By Name("Y"=w330, "dt"=w329) -> (w328:waveform(dbl))  [unwired: 1 in]
                    }
                    n134 = global read "Constants.vi" "Properties.Injector.Waveforms"() -> (w317:string)
                    n135 = call-poly <vilib>:"NI VeriStand - Set Item Property.vi"("error in (no error)"=w321, "Value"=w319, "Property Name"=w317, "Item Ref in"=w318) -> ("error out"=w320:errorcluster)  [unwired: 5 in, 2 out]
                    n136 = Build Array (concatenate)(w326, "Cursor.Reset") -> (w316:string[])
                  }
                  frame "Set Analysis Channels" {
                    n137 = property class="LstBox (strict)"(reference=w351, error in=w352) -> (error out=w345:errorcluster, "Item Names"=w350:string[], "Value"=w349:i32)  [unwired: 1 out]
                    n138 = call "Selection.Convert.Get.vi"("error in (no error)"=w345, "ListBox in"=w343) -> ("error out"=w344:errorcluster, "Analysis Options"=w342:T8)  [unwired: 8 in]
                    n139 = Index Array(array=w350, index=w349) -> (element=w339:string)
                    n140 = call <vilib>:"NI VeriStand - Get Item Ref by Relative Path.vi"("error in"=w344, "Relative Item Path"=w339, "Section Ref in"=w348) -> ("error out"=w347:errorcluster, "Item Ref"=w346:T5)  [unwired: 5 in, 2 out]
                    n141 = call "Analysis.Selection.Create.vi"("error in (no error)"=w347, "Name"=w339, "Analysis Options"=w342, "Item Ref in"=w346) -> ("error out"=w341:errorcluster)  [unwired: 7 in]
                  }
                  frame "Set Event Duration" {
                    n142 = global read "Constants.vi" "GlobalSettings.PreTrigger.Samples"() -> (w362:string)
                    n143 = property class="DigNum (strict)"(reference=w358, error in=w354) -> (error out=w359:errorcluster, "Value"=w357:u8)  [unwired: 1 out]
                    n144 = global read "Constants.vi" "GlobalSettings.InjectionDuration"() -> (w377:string)
                    n145 = global read "Constants.vi" "GlobalSettings.Name"() -> (w378:string)
                    n146 = global read "Constants.vi" "GlobalSettings.Name"() -> (w361:string)
                    n147 = Concatenate Strings(w378, "/" ("string"), w377) -> (w370:string)
                    n148 = Concatenate Strings(w361, "/" ("string"), w362) -> (w366:string)
                    n149 = call <vilib>:"NI VeriStand - Get Item Ref by Relative Path.vi"("error in"=w359, "Relative Item Path"=w366, "Section Ref in"=w360) -> ("error out"=w364:errorcluster, "Item Ref"=w365:T5)  [unwired: 5 in, 2 out]
                    n150 = call <vilib>:"NI VeriStand - Set Custom Device Channel Default Value.vi"("error in (no error)"=w364, "Default Value"=w357, "Channel Ref in"=w365) -> ("error out"=w353:errorcluster)  [unwired: 7 in, 1 out]
                    n151 = property class="DigNum (strict)"(reference=w375, error in=w353) -> (error out=w372:errorcluster, "Value"=w371:dbl)  [unwired: 1 out]
                    n152 = call <vilib>:"NI VeriStand - Get Item Ref by Relative Path.vi"("error in"=w372, "Relative Item Path"=w370, "Section Ref in"=w360) -> ("error out"=w374:errorcluster, "Item Ref"=w373:T5)  [unwired: 5 in, 2 out]
                    n153 = Multiply(x=w371, y=1000000.0) -> (x*y=w368:dbl)
                    n154 = call <vilib>:"NI VeriStand - Set Custom Device Channel Default Value.vi"("error in (no error)"=w374, "Default Value"=w368, "Channel Ref in"=w373) -> ("error out"=w355:errorcluster)  [unwired: 7 in, 1 out]
                  }
                }
              }
              event "Reset": Value Change {
                n155 = event-data() -> ()  [unwired: 2 out]
                n156 = Build Array (concatenate)(w383, "Tab.Update") -> (w382:string[])
              }
              event "Stages List": Value Change {
                n157 = event-data() -> ()  [unwired: 6 out]
                n158 = Build Array (concatenate)(w388, "Analysis.Update") -> (w386:string[])
              }
              event "Transitions": Value Change {
                n159 = event-data() -> ()  [unwired: 6 out]
                n160 = Build Array (concatenate)(w393, "Transitions.Update") -> (w392:string[])
              }
              event "Tab Control": Value Change {
                n161 = event-data() -> ()  [unwired: 7 out]
                n162 = Build Array (concatenate)(w398, "Tab.Update") -> (w397:string[])
              }
              event Value Change {
                n163 = event-data() -> ()  [unwired: 2 out]
                n164 = Unbundle By Name(w405) -> ("Pull In Transition"=w403:refnum<vi>)
                n165 = property class="Enum (strict)"(reference=w403, error in=w404) -> (error out=w402:errorcluster, "Value"=w401:T3)  [unwired: 1 out]
                n166 = case shown="\"Pull In Transition Pulses\"" w401 {
                  tunnel: w400 -> [w407 w410]
                  tunnel: [w406 w409] -> w399
                  frame "Pull In Transition Pulses" {
                    n167 = Build Array (concatenate)(w407, "Cursor.SetVoltage" ("string")) -> (w406:string[])
                  }
                  frame "Pull In Transition Current Drop" {
                    n168 = Build Array (concatenate)(w410, "Cursor.SetCurrent" ("string")) -> (w409:string[])
                  }
                }
              }
              event Value Change {
                n169 = event-data() -> ()  [unwired: 7 out]
                n170 = Unbundle By Name(w418) -> ("Stage Transition"=w416:refnum<vi>)
                n171 = property class="Enum (strict)"(reference=w416, error in=w417) -> (error out=w413:errorcluster, "Value"=w412:T4)  [unwired: 1 out]
                n172 = case shown="\"Stage Transition Active Time\"" w412 {
                  tunnel: w415 -> [w420 w423 w426 w429]
                  tunnel: [w419 w422 w425 w428] -> w414
                  frame "Stage Transition Voltage Increase" {
                    n173 = Build Array (concatenate)(w420, "Cursor.SetVoltage" ("string")) -> (w419:string[])
                  }
                  frame "Stage Transition Inactive Time" {
                    n174 = Build Array (concatenate)(w423, "Cursor.SetVoltage" ("string")) -> (w422:string[])
                  }
                  frame "Stage Transition Active Time" {
                    n175 = Build Array (concatenate)(w426, "Cursor.SetVoltage" ("string")) -> (w425:string[])
                  }
                  frame "Stage Transition Current Decrease" {
                    n176 = Build Array (concatenate)(w429, "Cursor.SetCurrent" ("string")) -> (w428:string[])
                  }
                }
              }
              event "Path": Value Change {
                n177 = event-data() -> ("NewVal"=w441:path)  [unwired: 1 out]
                n178 = Unbundle By Name(w431) -> ("Injection"=w437:refnum<vi>)
                n179 = call "Waveform.Selection.vi"("error in (no error)"=w440, "NewVal"=w441) -> ("error out"=w436:errorcluster, "Apply?"=w432:bool, "Data"=w438:waveform(dbl)[])  [unwired: 7 in]
                n180 = case shown="True" w432 {
                  tunnel: [w442 w446] -> w439
                  tunnel: w438 -> [_ w443]
                  tunnel: w437 -> [_ w445]
                  tunnel: w436 -> [w442 w444]
                  frame False {
                  }
                  frame True {
                    n181 = property class="WFGraph (strict)"(reference=w445, error in=w444, "Value"=w443) -> (error out=w446:errorcluster)  [unwired: 1 out]
                  }
                }
                n182 = Build Array (concatenate)(w435, string[] ["Path.Reset", "Cursor.Reset"]) -> (w434:string[])
              }
              event "Analysis": Shortcut Menu Selection (User) {
                n183 = event-data() -> ("ItemTag"=w448:string)  [unwired: 1 out]
                n184 = Unbundle By Name(w452) -> ("Analysis"=w451:refnum<vi>)
                n185 = case shown="\"Select All\"" w448 {
                  tunnel: [w455 w457] -> w449
                  tunnel: T8 {"Pull In Time"=FALSE, "Pull In Max Current"=FALSE, "Pull In Max Voltage"=FALSE, "Pull In Min Voltage"=FALSE, "Pull In Avg Voltage"=FALSE, "Hold Time"=FALSE, "Hold Max Current"=FALSE, "Hold Min Current"=FALSE, "Hold Avg Current"=FALSE, "Hold Max Voltage"=FALSE, "Hold Min Voltage"=FALSE, "Hold Avg Max Voltage"=FALSE, "Hold Avg Min Voltage"=FALSE, "Off Time"=FALSE, "Off Max Current"=FALSE, "Off Min Current"=FALSE, "Off Avg Current"=FALSE, "Off Max Voltage"=FALSE, "Off Min Voltage"=FALSE, "Off Avg Voltage"=FALSE, "Total Voltage Pulses"=FALSE, "Total Stage Time"=FALSE} ("Selections") -> [w455 w456]
                  frame "Deselect All", Default {
                  }
                  frame "Select All" {
                    n186 = Not(x=w456) -> (.not. x?=w457:T8)
                  }
                }
                n187 = call "Selection.Convert.Set.vi"("error in (no error)"=w453, "Selections"=w449, "ListBox in"=w451) -> ("error out"=w450:errorcluster)  [unwired: 8 in]
              }
              event "Pre-Trigger Samples", "Event Duration": Value Change {
                n188 = event-data() -> ()  [unwired: 7 out]
                n189 = Build Array (concatenate)(w462, "TotalDuration.Update") -> (w459:string[])
              }
              event "Injection": Scale Range Change {
                n190 = event-data() -> ()  [unwired: 9 out]
                n191 = Build Array (concatenate)(w467, "Cursor.Reset") -> (w464:string[])
              }
            }
          }
          frame "Analysis.Update" {
            n192 = Unbundle By Name(w472) -> ("Analysis"=w477:refnum<vi>, "Stages List"=w480:refnum<vi>)
            n193 = property class="LstBox (strict)"(reference=w480, error in=w470) -> (error out=w475:errorcluster, "Item Names"=w479:string[], "Value"=w478:i32)  [unwired: 1 out]
            n194 = Index Array(array=w479, index=w478) -> (element=w476:string)
            n195 = call <vilib>:"NI VeriStand - Get Item Ref by Relative Path.vi"("error in"=w475, "Relative Item Path"=w476, "Section Ref in"=w469) -> ("error out"=w474:errorcluster, "Item Ref"=w473:T5, "Found"=w468:bool)  [unwired: 5 in, 1 out]
            n196 = case shown="True" w468 {
              tunnel: w477 -> [_ w486]
              tunnel: w474 -> [w482 w485]
              tunnel: w473 -> [_ w484]
              tunnel: [w482 w483] -> w471
              frame False {
              }
              frame True {
                n197 = call "Analysis.Selection.Get.vi"("Action"=enum8{"Get", "Set"}."Get", "error in (no error)"=w485, "Item Ref in"=w484) -> ("error out"=w487:errorcluster, "Selections"=w488:T8)  [unwired: 6 in, 1 out]
                n198 = call "Selection.Convert.Set.vi"("error in (no error)"=w487, "Selections"=w488, "ListBox in"=w486) -> ("error out"=w483:errorcluster)  [unwired: 8 in]
              }
            }
          }
          frame "Cursor.Move" {
            n199 = Unbundle By Name(w504) -> ("Trigger Duration"=w496:refnum<vi>, "Level"=w506:refnum<vi>, "Pull In Transition"=w507:refnum<vi>, "Initial Voltage"=w508:refnum<vi>, "Event Duration"=w509:refnum<vi>, "Stage Transition"=w511:refnum<vi>, "Transitions"=w510:refnum<vi>, "Tab"=w516:refnum<vi>, "Injection"=w518:refnum<vi>)
            n200 = property class="WFGraph (strict)"(reference=w518, error in=w505) -> (error out=w517:errorcluster, "CrsrList"=w523:T12, "Value"=w502:waveform(dbl)[])  [unwired: 1 out]
            n201 = Index Array(array=w523) -> (element #1=w520:T13, element #2=w519:T13)  [unwired: 2 in]
            n202 = Unbundle By Name(w520) -> ("Position.X"=w500:dbl, "Position.Y"=w493:dbl)
            n203 = Unbundle By Name(w519) -> ("Position.X"=w499:dbl, "Position.Y"=w492:dbl)
            n204 = property class="TabCtl (strict)"(reference=w516, error in=w517) -> (error out=w515:errorcluster, "Value"=w514:T1)  [unwired: 1 out]
            n205 = Index Array(array=w502) -> (element=w501:waveform(dbl))  [unwired: 1 in]
            n206 = Subtract(x=w493, y=w492) -> (x-y=w521:dbl)
            n207 = Subtract(x=w500, y=w499) -> (x-y=w522:dbl)
            n208 = Max & Min(x=w493, y=w492) -> (max(x,y)=w490:dbl, min(x,y)=w491:dbl)
            n209 = Absolute Value(x=w521) -> (abs(x)=w513:dbl)
            n210 = Absolute Value(x=w522) -> (abs(x)=w512:dbl)
            n211 = case shown="\"Set Initial Voltage\"" w514 {
              tunnel: w515 -> [w530 w532 w542 w565]
              tunnel: [w527 w532 w539 w559] -> w503
              tunnel: w513 -> [_ _ w543 w564]
              tunnel: w512 -> [w529 _ w537 w562]
              tunnel: w511 -> [_ _ _ w561]
              tunnel: w510 -> [_ _ _ w563]
              tunnel: w509 -> [w528 _ _ _]
              tunnel: w508 -> [_ _ w541 _]
              tunnel: w507 -> [_ _ _ w556]
              tunnel: w506 -> [_ _ _ w557]
              tunnel: w501 -> [_ _ _ w555]
              tunnel: w500 -> [_ _ _ w554]
              tunnel: w499 -> [_ _ _ w553]
              tunnel: w498 -> [_ _ _ w549]
              tunnel: w497 -> [_ _ _ w548]
              tunnel: w496 -> [_ _ w538 _]
              tunnel: w495 -> [w526 w531 w536 w547]
              tunnel: [w525 w531 w536 w547] -> w494
              tunnel: w491 -> [_ _ w535 w546]
              tunnel: w490 -> [_ _ _ w545]
              frame "Set Event Duration" {
                n212 = property class="DigNum (strict)"(reference=w528, error in=w530, "Value"=w529) -> (error out=w527:errorcluster)  [unwired: 1 out]
                n213 = Build Array (concatenate)(w526, "TotalDuration.Update") -> (w525:string[])
              }
              frame Default {
              }
              frame "Set Initial Voltage" {
                n214 = Divide(x=w543, y=2.0) -> (x/y=w534:dbl)
                n215 = Add(x=w534, y=w535) -> (x+y=w533:dbl)
                n216 = property class="DigNum (strict)"(reference=w541, error in=w542, "Value"=w533) -> (error out=w540:errorcluster)  [unwired: 1 out]
                n217 = property class="DigNum (strict)"(reference=w538, error in=w540, "Value"=w537) -> (error out=w539:errorcluster)  [unwired: 1 out]
              }
              frame "Set Stage Parsing Parameters" {
                n218 = property class="LstBox (strict)"(reference=w563, error in=w565) -> (error out=w560:errorcluster, "Item Names"=w552:string[], "Value"=w551:i32)  [unwired: 1 out]
                n219 = Index Array(array=w552, index=w551) -> (element=w550:string)
                n220 = Quotient & Remainder(x=w551, y=w548) -> (x-y*floor(x/y)=w558:u32)  [unwired: 1 out]
                n221 = case shown="2" w558 {
                  tunnel: w564 -> [w576 w609 _ w624]
                  tunnel: w562 -> [_ w608 _ _]
                  tunnel: w561 -> [_ w607 _ _]
                  tunnel: w560 -> [w579 w606 w618 w626]
                  tunnel: [w575 w603 w618 w625] -> w559
                  tunnel: w557 -> [w574 w602 _ w622]
                  tunnel: w556 -> [w578 _ _ _]
                  tunnel: w555 -> [w572 _ _ _]
                  tunnel: w554 -> [w571 _ _ _]
                  tunnel: w553 -> [w570 _ _ _]
                  tunnel: w550 -> [w569 _ _ _]
                  tunnel: w549 -> [w566 _ _ _]
                  tunnel: w546 -> [_ w600 _ w621]
                  tunnel: w545 -> [_ w599 _ _]
                  frame 1 {
                    n222 = property class="Enum (strict)"(reference=w578, error in=w579) -> (error out=w568:errorcluster, "Value"=w577:T3)  [unwired: 1 out]
                    n223 = case shown="\"Pull In Transition Current Drop\"" w577 {
                      tunnel: [w593 w598] -> w573
                      tunnel: w576 -> [_ w598]
                      tunnel: w572 -> [w596 _]
                      tunnel: w571 -> [w595 _]
                      tunnel: w570 -> [w594 _]
                      tunnel: w569 -> [w591 _]
                      tunnel: w568 -> [w590 w597]
                      tunnel: [w583 w597] -> w567
                      tunnel: w566 -> [w588 _]
                      frame "Pull In Transition Pulses" {
                        n224 = Match Pattern(string=w591, regular expression="\\.") -> (before substring=w589:string)  [unwired: 1 in, 3 out]
                        n225 = call <vilib>:"NI VeriStand - Get Item Ref by Relative Path.vi"("error in"=w590, "Relative Item Path"=w589, "Section Ref in"=w588) -> ("error out"=w586:errorcluster, "Item Ref"=w587:T5)  [unwired: 5 in, 2 out]
                        n226 = call <vilib>:"NI VeriStand - Get Item Children.vi"("error in (no error)"=w586, "Item Ref in"=w587) -> ("error out"=w584:errorcluster, "Child Refs"=w585:T5[])  [unwired: 6 in, 2 out]
                        n227 = Index Array(array=w585) -> (element=w582:T5)  [unwired: 1 in]
                        n228 = call <vilib>:"NI VeriStand - Get Custom Device Channel Data.vi"("error in (no error)"=w584, "Channel Ref in"=w582) -> ("error out"=w583:errorcluster, "Channel"=w581:T14)  [unwired: 4 in, 4 out]
                        n229 = Unbundle By Name(w581) -> ("Default Value"=w580:dbl)
                        n230 = call "Pulses.Count.vi"("Dwell Limit"=w580, "X 2"=w594, "X"=w595, "Waveform"=w596) -> ("Numeric"=w593:i32)  [unwired: 7 in]
                      }
                      frame "Pull In Transition Current Drop" {
                      }
                    }
                    n231 = property class="DigNum (strict)"(reference=w574, error in=w567, "Value"=w573) -> (error out=w575:errorcluster)  [unwired: 1 out]
                  }
                  frame 2 {
                    n232 = property class="Enum (strict)"(reference=w607, error in=w606) -> (error out=w604:errorcluster, "Value"=w605:T4)  [unwired: 1 out]
                    n233 = case shown="\"Stage Transition Voltage Increase\"" w605 {
                      tunnel: [w610 w611 w615 w617] -> w601
                      tunnel: w609 -> [_ _ w613 w617]
                      tunnel: w608 -> [w610 w611 _ _]
                      tunnel: w600 -> [_ _ w614 _]
                      tunnel: w599 -> [_ _ _ _]
                      frame "Stage Transition Inactive Time" {
                      }
                      frame "Stage Transition Active Time" {
                      }
                      frame "Stage Transition Voltage Increase" {
                        n234 = Divide(x=w613, y=2.0) -> (x/y=w616:dbl)
                        n235 = Add(x=w616, y=w614) -> (x+y=w615:dbl)
                      }
                      frame "Stage Transition Current Decrease" {
                      }
                    }
                    n236 = property class="DigNum (strict)"(reference=w602, error in=w604, "Value"=w601) -> (error out=w603:errorcluster)  [unwired: 1 out]
                  }
                  frame Default {
                  }
                  frame 0 {
                    n237 = Divide(x=w624, y=2.0) -> (x/y=w620:dbl)
                    n238 = Add(x=w620, y=w621) -> (x+y=w619:dbl)
                    n239 = property class="DigNum (strict)"(reference=w622, error in=w626, "Value"=w619) -> (error out=w625:errorcluster)  [unwired: 1 out]
                  }
                }
              }
            }
          }
          frame "Cursor.Reset" {
            n240 = Unbundle By Name(w640) -> ("Injection"=w639:refnum<vi>)
            n241 = property class="WFGraph (strict)"(reference=w639, error in=w632) -> (reference out=w637:refnum<vi>, error out=w638:errorcluster, "CrsrList"=w636:T12, "Value"=w628:waveform(dbl)[], "XScale.Minimum"=w629:dbl)
            n242 = Index Array(array=w628) -> (element=w631:waveform(dbl))  [unwired: 1 in]
            n243 = Unbundle By Name(w631) -> ("dt"=w630:dbl)
            n244 = Divide(x=w629, y=w630) -> (x/y=w627:dbl)
            n245 = for {
              tunnel: w636 -> [w643] mode=indexing
              tunnel: [w642] -> w635 mode=indexing
              tunnel: w627 -> [w641]
              n246 = Bundle By Name(cluster=w643, "Index"=w641) -> (w642:T13)
            }
            n247 = property class="WFGraph (strict)"(reference=w637, error in=w638, "CrsrList"=w635) -> (error out=w633:errorcluster)  [unwired: 1 out]
          }
          frame "Cursor.SetCurrent" {
            n248 = Unbundle By Name(w647) -> ("Injection"=w646:refnum<vi>)
            n249 = property class="WFGraph (strict)"(reference=w646, error in=w645) -> (reference out=w648:refnum<vi>, error out=w651:errorcluster, "CrsrList"=w652:T12)
            n250 = for {
              tunnel: w652 -> [w657] mode=indexing
              shift-right: [w656] -> w650
              shift-left: w651 -> [w656]
              tunnel: [w655] -> w649 mode=indexing
              n251 = Bundle By Name(cluster=w657, "Plot"=1) -> (w655:T13)
            }
            n252 = property class="WFGraph (strict)"(reference=w648, error in=w650, "CrsrList"=w649) -> (error out=w644:errorcluster)  [unwired: 1 out]
          }
          frame "Cursor.SetVoltage" {
            n253 = Unbundle By Name(w661) -> ("Injection"=w660:refnum<vi>)
            n254 = property class="WFGraph (strict)"(reference=w660, error in=w659) -> (reference out=w662:refnum<vi>, error out=w665:errorcluster, "CrsrList"=w666:T12)
            n255 = for {
              tunnel: w666 -> [w671] mode=indexing
              shift-right: [w670] -> w664
              shift-left: w665 -> [w670]
              tunnel: [w669] -> w663 mode=indexing
              n256 = Bundle By Name(cluster=w671, "Plot"=0) -> (w669:T13)
            }
            n257 = property class="WFGraph (strict)"(reference=w662, error in=w664, "CrsrList"=w663) -> (error out=w658:errorcluster)  [unwired: 1 out]
          }
          frame "Graph.Load" {
            w675 = waveform(dbl)[] []
            n258 = global read "Constants.vi" "Properties.Injector.Waveforms"() -> (w683:string)
            n259 = call-poly <vilib>:"NI VeriStand - Get Item Property.vi"("error in (no error)"=w676, "Default Value"=w675, "Property Name"=w683, "Item Ref in"=w677) -> ("error out"=w680:errorcluster, "Value"=w678:variant, "Found?"=w681:bool)  [unwired: 4 in, 1 out]
            n260 = case shown="True" w681 {
              tunnel: w675 -> [w686 w689]
              tunnel: [w686 w687] -> w674
              tunnel: w680 -> [w685 w691]
              tunnel: [w685 w690] -> w679
              tunnel: w678 -> [_ w688]
              frame False {
              }
              frame True {
                n261 = Variant To Data(error in=w691, type=w689, Variant=w688) -> (data=w687:waveform(dbl)[], error out=w690:errorcluster)
              }
            }
            n262 = Unbundle By Name(w684) -> ("Injection"=w682:refnum<vi>)
            n263 = property class="WFGraph (strict)"(reference=w682, error in=w679, "Value"=w674) -> (error out=w673:errorcluster)  [unwired: 1 out]
          }
          frame "EventDuration.Update" {
            n264 = global read "Constants.vi" "GlobalSettings.PreTrigger.Samples"() -> (w699:string)
            n265 = global read "Constants.vi" "GlobalSettings.InjectionDuration"() -> (w721:string)
            n266 = global read "Constants.vi" "GlobalSettings.Name"() -> (w722:string)
            n267 = global read "Constants.vi" "GlobalSettings.Name"() -> (w698:string)
            n268 = Concatenate Strings(w722, "/" ("string"), w721) -> (w719:string)
            n269 = Concatenate Strings(w698, "/" ("string"), w699) -> (w701:string)
            n270 = call <vilib>:"NI VeriStand - Get Item Ref by Relative Path.vi"("error in"=w716, "Relative Item Path"=w719, "Section Ref in"=w693) -> ("error out"=w718:errorcluster, "Item Ref"=w717:T5, "Section Ref out"=w692:T5)  [unwired: 5 in, 1 out]
            n271 = call <vilib>:"NI VeriStand - Get Custom Device Channel Data.vi"("error in (no error)"=w718, "Channel Ref in"=w717) -> ("error out"=w713:errorcluster, "Channel"=w712:T14)  [unwired: 4 in, 4 out]
            n272 = Unbundle By Name(w712) -> ("Default Value"=w711:dbl)
            n273 = Unbundle By Name(w715) -> ("Pre-Trigger Samples"=w695:refnum<vi>, "Event Duration"=w714:refnum<vi>)
            n274 = Divide(x=w711, y=1000000.0 ("x")) -> (x/y=w710:dbl)
            n275 = property class="DigNum (strict)"(reference=w714, error in=w713, "Value"=w710) -> (error out=w697:errorcluster)  [unwired: 1 out]
            n276 = Build Array (concatenate)(w707, "Cursor.SetVoltage" ("string")) -> (w706:string[])
            n277 = call <vilib>:"NI VeriStand - Get Item Ref by Relative Path.vi"("error in"=w697, "Relative Item Path"=w701, "Section Ref in"=w692) -> ("error out"=w702:errorcluster, "Item Ref"=w703:T5)  [unwired: 5 in, 2 out]
            n278 = call <vilib>:"NI VeriStand - Get Custom Device Channel Data.vi"("error in (no error)"=w702, "Channel Ref in"=w703) -> ("error out"=w704:errorcluster, "Channel"=w705:T14)  [unwired: 4 in, 4 out]
            n279 = Unbundle By Name(w705) -> ("Default Value"=w694:dbl)
            n280 = property class="DigNum (strict)"(reference=w695, error in=w704, "Value"=w694) -> (error out=w696:errorcluster)  [unwired: 1 out]
          }
          frame "InitialVoltage.Update" {
            n281 = global read "Constants.vi" "GlobalSettings.InitialVoltageThreshold"() -> (w765:string)
            n282 = global read "Constants.vi" "GlobalSettings.Filter.Duration"() -> (w746:string)
            n283 = global read "Constants.vi" "GlobalSettings.ActiveEdge"() -> (w737:string)
            n284 = global read "Constants.vi" "GlobalSettings.Name"() -> (w766:string)
            n285 = global read "Constants.vi" "GlobalSettings.Name"() -> (w745:string)
            n286 = global read "Constants.vi" "GlobalSettings.Name"() -> (w738:string)
            n287 = Build Array (concatenate)(w767, "Cursor.SetVoltage" ("string")) -> (w754:string[])
            n288 = Concatenate Strings(w766, "/" ("string"), w765) -> (w763:string)
            n289 = Concatenate Strings(w745, "/" ("string"), w746) -> (w748:string)
            n290 = Concatenate Strings(w738, "/" ("string"), w737) -> (w727:string)
            n291 = call <vilib>:"NI VeriStand - Get Item Ref by Relative Path.vi"("error in"=w760, "Relative Item Path"=w763, "Section Ref in"=w744) -> ("error out"=w762:errorcluster, "Item Ref"=w761:T5, "Section Ref out"=w739:T5)  [unwired: 5 in, 1 out]
            n292 = call <vilib>:"NI VeriStand - Get Custom Device Channel Data.vi"("error in (no error)"=w762, "Channel Ref in"=w761) -> ("error out"=w757:errorcluster, "Channel"=w756:T14)  [unwired: 4 in, 4 out]
            n293 = Unbundle By Name(w759) -> ("Active Edge"=w735:refnum<vi>, "Trigger Duration"=w743:refnum<vi>, "Initial Voltage"=w758:refnum<vi>)
            n294 = Unbundle By Name(w756) -> ("Default Value"=w755:dbl)
            n295 = property class="DigNum (strict)"(reference=w758, error in=w757, "Value"=w755) -> (error out=w733:errorcluster)  [unwired: 1 out]
            n296 = call <vilib>:"NI VeriStand - Get Item Ref by Relative Path.vi"("error in"=w733, "Relative Item Path"=w748, "Section Ref in"=w739) -> ("error out"=w749:errorcluster, "Item Ref"=w750:T5, "Section Ref out"=w728:T5)  [unwired: 5 in, 1 out]
            n297 = call <vilib>:"NI VeriStand - Get Custom Device Channel Data.vi"("error in (no error)"=w749, "Channel Ref in"=w750) -> ("error out"=w751:errorcluster, "Channel"=w752:T14)  [unwired: 4 in, 4 out]
            n298 = Unbundle By Name(w752) -> ("Default Value"=w741:dbl)
            n299 = Divide(x=w741, y=1000000.0 ("x")) -> (x/y=w740:dbl)
            n300 = property class="DigNum (strict)"(reference=w743, error in=w751, "Value"=w740) -> (error out=w729:errorcluster)  [unwired: 1 out]
            n301 = call <vilib>:"NI VeriStand - Get Item Ref by Relative Path.vi"("error in"=w729, "Relative Item Path"=w727, "Section Ref in"=w728) -> ("error out"=w732:errorcluster, "Item Ref"=w731:T5)  [unwired: 5 in, 2 out]
            n302 = call <vilib>:"NI VeriStand - Get Custom Device Channel Data.vi"("error in (no error)"=w732, "Channel Ref in"=w731) -> ("error out"=w726:errorcluster, "Channel"=w730:T14)  [unwired: 4 in, 4 out]
            n303 = Unbundle By Name(w730) -> ("Default Value"=w725:dbl)
            n304 = To Long Integer(number=w725) -> (32bit integer=w724:i32)
            n305 = Greater Than 0?(x=w724) -> (x > 0?=w723:bool)
            n306 = property class="Bool (strict)"(reference=w735, error in=w726, "Value"=w723) -> (error out=w734:errorcluster)  [unwired: 1 out]
          }
          frame "Stages.Update" {
            n307 = global read "Constants.vi" "Properties.MaxShots"() -> (w777:string)
            n308 = call-poly <vilib>:"NI VeriStand - Get Item Property.vi"("error in (no error)"=w776, "Default Value"=u32 1, "Property Name"=w777, "Item Ref in"=w774) -> ("error out"=w775:errorcluster, "Value"=w769:u32, "Item Ref out"=w773:T5)  [unwired: 4 in, 1 out]
            n309 = global read "Constants.vi" "GUID.Analysis Stage"() -> (w779:string)
            n310 = call-poly <vilib>:"NI VeriStand - Search for Item.vi"("error in"=w775, "Item GUID"=w779, "Section Ref in"=w773) -> ("error out"=w793:errorcluster, "Item Refs"=w778:T5[])  [unwired: 5 in, 2 out]
            n311 = Unbundle By Name(w791) -> ("Max Shots"=w772:refnum<vi>, "Transitions"=w784:refnum<vi>, "Stages List"=w789:refnum<vi>, "Stages"=w790:refnum<vi>)
            n312 = for {
              tunnel: w778 -> [w803] mode=indexing
              shift-right: [w801] -> w792
              shift-left: w793 -> [w804]
              tunnel: [w800] -> w786 mode=indexing
              n313 = call <vilib>:"NI VeriStand - Get Item Data.vi"("error in (no error)"=w804, "Item Ref in"=w803) -> ("error out"=w801:errorcluster, "Item Info"=w802:T16)  [unwired: 6 in, 2 out]
              n314 = Unbundle By Name(w802) -> ("Name"=w800:string)
            }
            n315 = property class="Arr (strict)"(reference=w790, error in=w792, "Value"=w786) -> (error out=w788:errorcluster)  [unwired: 1 out]
            n316 = for {
              tunnel: w786 -> [w795] mode=indexing
              tunnel: string[] [".Voltage Threshold", ".Pull In Settings", ".Transition Settings"] -> [w796]
              tunnel: [w794] -> w782 mode=concatenating
              n317 = for {
                tunnel: w796 -> [w799] mode=indexing
                tunnel: w795 -> [w798]
                tunnel: [w797] -> w794 mode=indexing
                n318 = Concatenate Strings(w798, w799) -> (w797:string)
              }
            }
            n319 = property class="LstBox (strict)"(reference=w789, error in=w788, "Item Names"=w786, "Value"=0 ("Value (Signaling)")) -> (error out=w783:errorcluster)  [unwired: 1 out]
            n320 = property class="LstBox (strict)"(reference=w784, error in=w783, "Item Names"=w782, "Value"=0 ("Value (Signaling)")) -> (error out=w771:errorcluster)  [unwired: 1 out]
            n321 = property class="Enum (strict)"(reference=w772, error in=w771, "Value"=w769) -> (error out=w770:errorcluster)  [unwired: 1 out]
          }
          frame "Tab.Update" {
            n322 = Unbundle By Name(w805) -> ("Step"=w808:refnum<vi>, "Tab"=w810:refnum<vi>)
            n323 = property class="TabCtl (strict)"(reference=w810, error in=w811) -> (error out=w816:errorcluster, "Pages"=w815:refnum<vi>[], "Value"=w812:T1)  [unwired: 1 out]
            n324 = for {
              tunnel: w815 -> [w822] mode=indexing
              tunnel: [w821] -> w814 mode=indexing
              shift-right: [w820] -> w809
              shift-left: w816 -> [w823]
              n325 = property class="Page"(reference=w822, error in=w823) -> (error out=w820:errorcluster, "PageLabel"=w821:string)  [unwired: 1 out]
            }
            n326 = Index Array(array=w814, index=w812) -> (element=w813:string)
            n327 = property class="Str"(reference=w808, error in=w809, "Value"=w813) -> (error out=w807:errorcluster)  [unwired: 1 out]
            n328 = case shown="\"Set Stage Parsing Parameters\"" w812 {
              tunnel: w807 -> [w828 w833 w838 w843 w845 w850]
              tunnel: [w828 w833 w838 w843 w845 w850] -> w819
              tunnel: [w826 w831 w836 w841 w846 w851] -> w818
              tunnel: w817 -> [w827 w830 w837 w842 w847 w852]
              tunnel: [w824 w829 w834 w839 w844 w849] -> w806
              tunnel: w805 -> [w824 w829 w834 w839 w844 w849]
              frame "Set Shots and Stages" {
                n329 = Build Array (concatenate)(w827, string[] ["Stages.Update"]) -> (w826:string[])
              }
              frame "Load Waveform" {
                n330 = Build Array (concatenate)(w830, string[] ["Graph.Load", "Cursor.Reset", "Path.Reset"]) -> (w831:string[])
              }
              frame "Set Stage Parsing Parameters" {
                n331 = Build Array (concatenate)(w837, string[] ["Transitions.Update"]) -> (w836:string[])
              }
              frame "Set Analysis Channels" {
                n332 = Build Array (concatenate)(w842, string[] ["Analysis.Update"]) -> (w841:string[])
              }
              frame "Set Event Duration" {
                n333 = Build Array (concatenate)(w847, string[] ["EventDuration.Update", "TotalDuration.Update"]) -> (w846:string[])
              }
              frame "Set Initial Voltage" {
                n334 = Build Array (concatenate)(w852, string[] ["InitialVoltage.Update"]) -> (w851:string[])
              }
            }
          }
          frame "TotalDuration.Update" {
            n335 = Unbundle By Name(w866) -> ("Total Duration"=w857:refnum<vi>, "Event Duration"=w863:refnum<vi>, "Pre-Trigger Samples"=w865:refnum<vi>, "dt"=w861:dbl)
            n336 = property class="DigNum (strict)"(reference=w865, error in=w855) -> (error out=w864:errorcluster, "Value"=w862:u8)  [unwired: 1 out]
            n337 = Multiply(x=w862, y=w861) -> (x*y=w859:dbl)
            n338 = property class="DigNum (strict)"(reference=w863, error in=w864) -> (error out=w858:errorcluster, "Value"=w860:dbl)  [unwired: 1 out]
            n339 = Add(x=w860, y=w859) -> (x+y=w856:dbl)
            n340 = property class="DigNum (strict)"(reference=w857, error in=w858, "Value"=w856) -> (error out=w854:errorcluster)  [unwired: 1 out]
          }
          frame "Transitions.Update" {
            n341 = Unbundle By Name(w868) -> ("Level"=w879:refnum<vi>, "Pull In Transition"=w881:refnum<vi>, "Stage Transition"=w882:refnum<vi>, "Transitions"=w883:refnum<vi>)
            n342 = property class="LstBox (strict)"(reference=w883, error in=w878) -> (error out=w875:errorcluster, "Item Names"=w872:string[], "Value"=w880:i32)  [unwired: 1 out]
            n343 = Empty Array?(array=w872) -> (empty?=w870:bool)
            n344 = case shown="False" w870 {
              tunnel: w882 -> [w903 _]
              tunnel: w881 -> [w902 _]
              tunnel: w880 -> [w897 _]
              tunnel: w879 -> [w895 _]
              tunnel: w877 -> [w894 _]
              tunnel: [w893 w1005] -> w876
              tunnel: w875 -> [w891 w1005]
              tunnel: w874 -> [w889 w1004]
              tunnel: [w888 w1004] -> w873
              tunnel: w872 -> [w887 _]
              tunnel: w871 -> [w886 _]
              tunnel: [w885 w1003] -> w869
              tunnel: w868 -> [w884 w1003]
              frame False {
                n345 = Quotient & Remainder(x=w897, y=w886) -> (x-y*floor(x/y)=w896:u32)  [unwired: 1 out]
                n346 = Index Array(array=w887, index=w897) -> (element=w898:string)
                n347 = Match Pattern(string=w898, regular expression="\\.") -> (before substring=w900:string)  [unwired: 1 in, 3 out]
                n348 = call <vilib>:"NI VeriStand - Get Item Ref by Relative Path.vi"("error in"=w891, "Relative Item Path"=w900, "Section Ref in"=w894) -> ("error out"=w890:errorcluster, "Item Ref"=w901:T5, "Found"=w892:bool)  [unwired: 5 in, 1 out]
                n349 = case shown="False" w892 {
                  tunnel: w903 -> [_ w919]
                  tunnel: w902 -> [_ w918]
                  tunnel: w901 -> [_ w916]
                  tunnel: w890 -> [w906 w915]
                  tunnel: w896 -> [_ w914]
                  tunnel: w895 -> [_ w913]
                  tunnel: [w906 w912] -> w893
                  tunnel: w889 -> [w905 w910]
                  tunnel: [w905 w909] -> w888
                  tunnel: [w904 w908] -> w885
                  tunnel: w884 -> [w904 w907]
                  frame False {
                  }
                  frame True {
                    n350 = call <vilib>:"NI VeriStand - Get Item Children.vi"("error in (no error)"=w915, "Item Ref in"=w916) -> ("error out"=w911:errorcluster, "Child Refs"=w917:T5[])  [unwired: 6 in, 2 out]
                    n351 = case shown="0" w914 {
                      selector: w914 -> [w932 w952 w983 _]
                      tunnel: w919 -> [w938 w963 w974 _]
                      tunnel: w918 -> [w937 w962 w975 _]
                      tunnel: [w927 w946 w977 w1002] -> w912
                      tunnel: w917 -> [w936 w961 w991 _]
                      tunnel: w911 -> [w930 w950 w981 w1002]
                      tunnel: w913 -> [w929 w948 w979 _]
                      tunnel: w910 -> [w921 w943 w969 w1001]
                      tunnel: [w922 w942 w968 w1001] -> w909
                      tunnel: [w920 w939 w966 w1000] -> w908
                      tunnel: w907 -> [w920 w939 w966 w1000]
                      frame 0 {
                        n352 = Index Array(array=w936, index=w932) -> (element=w931:T5)
                        n353 = property class="Enum (strict)"(reference=w938, error in=w930, "Visible"=FALSE) -> (error out=w933:errorcluster)  [unwired: 1 out]
                        n354 = call <vilib>:"NI VeriStand - Get Custom Device Channel Data.vi"("error in (no error)"=w933, "Channel Ref in"=w931) -> ("error out"=w924:errorcluster, "Channel"=w926:T14)  [unwired: 4 in, 4 out]
                        n355 = Unbundle By Name(w926) -> ("Default Value"=w925:dbl)
                        n356 = property class="Enum (strict)"(reference=w937, error in=w924, "Visible"=FALSE) -> (error out=w928:errorcluster)  [unwired: 1 out]
                        n357 = Build Array (concatenate)(w921, "Cursor.SetVoltage" ("string")) -> (w922:string[])
                        n358 = property class="DigNum (strict)"(reference=w929, error in=w928, "Value"=w925) -> (error out=w927:errorcluster)  [unwired: 1 out]
                      }
                      frame 1 {
                        w955 = Stage.PullIn.Types."Pull In Transition Pulses" ("Value")
                        n359 = Index Array(array=w961, index=w952) -> (element=w951:T5)
                        n360 = property class="Enum (strict)"(reference=w963, error in=w950, "Visible"=FALSE) -> (error out=w954:errorcluster)  [unwired: 1 out]
                        n361 = call <vilib>:"NI VeriStand - Get Custom Device Channel Data.vi"("error in (no error)"=w954, "Channel Ref in"=w951) -> ("error out"=w957:errorcluster, "Channel"=w945:T14, "Channel Name"=w949:string)  [unwired: 4 in, 3 out]
                        n362 = Unbundle By Name(w945) -> ("Default Value"=w944:dbl)
                        n363 = call <userlib>:"Set Enum String Value__ogtk.vi"("error in (no error)"=w957, "String Value"=w949, "Default Enum Value"=w955) -> ("error out"=w958:errorcluster, "Enum"=w959:variant)  [unwired: 7 in]
                        n364 = Variant To Data(error in=w958, type=w955, Variant=w959) -> (data=w940:T3, error out=w953:errorcluster)
                        n365 = case shown="\"Pull In Transition Current Drop\"" w940 {
                          tunnel: ["Cursor.SetCurrent" ("string") "Cursor.SetVoltage" ("string")] -> w941
                          frame "Pull In Transition Current Drop" {
                          }
                          frame "Pull In Transition Pulses" {
                          }
                        }
                        n366 = property class="Enum (strict)"(reference=w962, error in=w953, "Value"=w940, "Visible"=TRUE) -> (error out=w947:errorcluster)  [unwired: 1 out]
                        n367 = property class="DigNum (strict)"(reference=w948, error in=w947, "Value"=w944) -> (error out=w946:errorcluster)  [unwired: 1 out]
                        n368 = Build Array (concatenate)(w943, w941) -> (w942:string[])
                      }
                      frame 2 {
                        w973 = Stage.Transition.Types."Stage Transition Inactive Time" ("Value")
                        n369 = Index Array(array=w991, index=w983) -> (element=w982:T5)
                        n370 = property class="Enum (strict)"(reference=w975, error in=w981, "Visible"=FALSE) -> (error out=w985:errorcluster)  [unwired: 1 out]
                        n371 = call <vilib>:"NI VeriStand - Get Custom Device Channel Data.vi"("error in (no error)"=w985, "Channel Ref in"=w982) -> ("error out"=w987:errorcluster, "Channel"=w976:T14, "Channel Name"=w980:string)  [unwired: 4 in, 3 out]
                        n372 = Unbundle By Name(w976) -> ("Default Value"=w971:dbl)
                        n373 = call <userlib>:"Set Enum String Value__ogtk.vi"("error in (no error)"=w987, "String Value"=w980, "Default Enum Value"=w973) -> ("error out"=w988:errorcluster, "Enum"=w989:variant)  [unwired: 7 in]
                        n374 = Variant To Data(error in=w988, type=w973, Variant=w989) -> (data=w967:T4, error out=w984:errorcluster)
                        n375 = case shown="\"Stage Transition Inactive Time\", \"Stage Transition Active Time\"" w967 {
                          tunnel: [w997 w999] -> w972
                          tunnel: w971 -> [w998 w999]
                          frame "Stage Transition Inactive Time", "Stage Transition Active Time" {
                            n376 = Divide(x=w998, y=1000000.0) -> (x/y=w997:dbl)
                          }
                          frame Default {
                          }
                        }
                        n377 = case shown="\"Stage Transition Active Time\"" w967 {
                          tunnel: ["Cursor.SetVoltage" ("string") "Cursor.SetCurrent" ("string") "Cursor.SetVoltage" ("string") "Cursor.SetVoltage" ("string")] -> w970
                          frame "Stage Transition Voltage Increase" {
                          }
                          frame "Stage Transition Current Decrease" {
                          }
                          frame "Stage Transition Inactive Time" {
                          }
                          frame "Stage Transition Active Time" {
                          }
                        }
                        n378 = property class="Enum (strict)"(reference=w974, error in=w984, "Value"=w967, "Visible"=TRUE) -> (error out=w978:errorcluster)  [unwired: 1 out]
                        n379 = property class="DigNum (strict)"(reference=w979, error in=w978, "Value"=w972) -> (error out=w977:errorcluster)  [unwired: 1 out]
                        n380 = Build Array (concatenate)(w969, w970) -> (w968:string[])
                      }
                      frame Default {
                      }
                    }
                  }
                }
              }
              frame True {
              }
            }
          }
          frame "UI.Initialize" {
            w1026 = waveform(dbl)[] []
            n381 = global read "Constants.vi" "Properties.Injector.Waveforms"() -> (w1036:string)
            n382 = call-poly <vilib>:"NI VeriStand - Get Item Property.vi"("error in (no error)"=w1029, "Default Value"=w1026, "Property Name"=w1036, "Item Ref in"=w1022) -> ("error out"=w1033:errorcluster, "Value"=w1031:variant, "Found?"=w1034:bool)  [unwired: 4 in, 1 out]
            n383 = case shown="False" w1034 {
              tunnel: w1026 -> [w1040 w1045]
              tunnel: [w1040 w1042] -> w1025
              tunnel: w1033 -> [w1039 w1047]
              tunnel: [w1039 w1046] -> w1032
              tunnel: w1031 -> [_ w1044]
              tunnel: [0 1] -> w1028
              tunnel: [T7."Disabled and Grayed Out" ("Disabled") T7."Enabled" ("Disabled")] -> w1007
              frame False {
              }
              frame True {
                n384 = Variant To Data(error in=w1047, type=w1045, Variant=w1044) -> (data=w1042:waveform(dbl)[], error out=w1046:errorcluster)
              }
            }
            n385 = Unbundle By Name(w1015) -> ("Next"=w1009:refnum<vi>, "Back"=w1010:refnum<vi>, "Tab"=w1030:refnum<vi>, "Injection"=w1035:refnum<vi>)
            n386 = property class="WFGraph (strict)"(reference=w1035, error in=w1032, "Value"=w1025) -> (error out=w1024:errorcluster)  [unwired: 1 out]
            n387 = property class="TabCtl (strict)"(reference=w1030, error in=w1024, "Value"=w1028) -> (error out=w1012:errorcluster)  [unwired: 1 out]
            n388 = property class="Bool"(reference=w1010, error in=w1012, "DisabledEnum"=w1007) -> (error out=w1013:errorcluster)  [unwired: 1 out]
            n389 = property class="Bool"(reference=w1009, error in=w1013, "DisabledEnum"=T7."Enabled" ("Disabled")) -> (error out=w1011:errorcluster)  [unwired: 1 out]
            n390 = global read "Constants.vi" "GUID.MeasurementType"() -> (w1021:string)
            n391 = call-poly <vilib>:"NI VeriStand - Search for Item.vi"("Direction (Down)"=Search_Direction."Up", "error in"=w1011, "Item GUID"=w1021, "Section Ref in"=w1022) -> ("error out"=w1019:errorcluster, "Item Ref"=w1020:T5)  [unwired: 4 in, 2 out]
            n392 = call "Measurement Type FG.vi"("Action"=enum8{"GET", "SET"}."GET", "error in (no error)"=w1019, "Item Ref"=w1020) -> ("error out"=w1018:errorcluster, "Sample rate (S/s)"=w1006:u32)  [unwired: 6 in, 1 out]
            n393 = Reciprocal(x=w1006) -> (1/x=w1016:dbl)
            n394 = Bundle By Name(cluster=w1015, "dt"=w1016) -> (w1014:T6)
          }
          frame Default {
          }
          frame "Path.Reset" {
            n395 = Unbundle By Name(w1054) -> ("Path"=w1052:refnum<vi>)
            n396 = property class="Path"(reference=w1052, error in=w1056, "Value"=path "") -> (error out=w1053:errorcluster)  [unwired: 1 out]
          }
        }
        n397 = call <vilib>:"Simple Error Handler.vi"("error in (no error)"=w52) -> ("error out"=w51:errorcluster)  [unwired: 1 in, 7 out]
        n398 = call <vilib>:"Clear Errors.vi"("error in (no error)"=w51) -> ("error out"=w50:errorcluster)  [unwired: 1 in, 5 out]
      }
      n399 = Unregister For Events(event registration refnum=w31, error in=w39) -> (error out=w38:errorcluster)
    }
    frame Error {
      n400 = call <vilib>:"Simple Error Handler.vi"("error in (no error)"=w1059) -> ("error out"=w1058:errorcluster)  [unwired: 1 in, 7 out]
      n401 = call <vilib>:"Clear Errors.vi"("error in (no error)"=w1058) -> ("error out"=w1057:errorcluster)  [unwired: 1 in, 5 out]
    }
  }
  n402 = invoke class="VI" method="FP.Close"(error in=w29) -> (error out=w28:errorcluster)  [unwired: 2 in, 2 out]
  n403 = call <vilib>:"NI VeriStand - Signal When Ready for Shutdown.vi"("error in (no error)"=w28) -> ("error out"=→"error out":errorcluster)  [unwired: 10 out]
